vi "ScannerControl.vi"() -> ()   [LabVIEW 2020]
uses:
  <vilib>/Math Plots/3D Math Plots/3D Scatter/3D Scatter XCtrl/3D Scatter.xctl
  <vilib>/userDefined/High Color/IMAQdx.ctl
  <vilib>/vision/Image Controls.llb/IMAQ Image.ctl
  SubVI/GRBL/Status.ctl
  <vilib>/event_ctls.llb/usereventprio.ctl
  <vilib>/vision/driver/IMAQdx.llb/IMAQdx Buffer Number Mode.ctl
  <vilib>/Math Plots/3D Math Plots/3D Scatter/3D Scatter Datatype/Public/Plot Helper (Vector).vi
  <vilib>/Instr/_visa.llb/VISA Configure Serial Port (Instr).vi
  <vilib>/ErrorRing/Error Ring.xnode
  SubVI/GRBL/GRBL 1.1.lvlib
  <vilib>/Math Plots/3D Math Plots/3D Scatter/3D Scatter Datatype/3D Scatter Datatype.lvclass
  <vilib>/vision/driver/NI_Vision_Acquisition_Software.lvlib
panel:
  out "LocationPollingStart":u32
  out "error out":errorcluster
  in  "Save Button":bool
  out "Sys Status":T1
  out "dt polling (ms)":dbl
  out "X encoder count":dbl format="%.2f"
  out "Z Distance(mm)":dbl
  out "X (mm)":dbl
  in  "3DProfileScan":bool
  in  "Pre Scan Speed (mm/min)":sgl=3000.0
  in  "Y Pixel Size(mm)":dbl=1.0
  in  "Y distance(mm)":dbl=10.0
  in  "X distance (mm)":dbl=10.0
  in  "Range Finder COM":refnum<visa-resource-name>="COM5"
  in  "Stage COM port":refnum<visa-resource-name>="COM4"
  in  "ShowFLImIntensity":bool
  in  "Upper Z limite(mm)":dbl=10.0
  in  "Remove Z outlier":bool
  in  "Probe Radius(2mm)":dbl=2.0 format="%#_13g"
  in  "Interpolate Scan":bool
  in  "FollowScanGridSize(mm)":dbl=2.0 format="%#_13g"
  in  "Calc follow scan":bool
  in  "Follow Z offset(mm)":dbl=1.0
  out "3D Profile":refnum<class "3D Plot Datatype.lvclass">[](xcontrol)
  in  "Follow Speed (mm/min)":sgl=3000.0
  in  "Follow Scan":bool
  in  "Plot 3D":bool
  in  "Tab Control":T2(tab)
  out "Scan Origin MPos":cluster{"X":sgl, "Y":sgl, "Z":sgl}
  in  "Set Origin":bool
  in  "Jog Step Size(mm)":dbl=5.0
  in  "Z--":bool
  in  "Z++":bool
  in  "Y--":bool
  in  "Y++":bool
  in  "X--":bool
  in  "X++":bool
  in  "Hault":bool
  in  "Home":bool
  in  "GoToZero":bool
  out "Current Machine Pos":cluster{"X":sgl, "Y":sgl, "Z":sgl}
  in  "Poll grbl position?":bool
  out "Stage Home MPos":cluster{"X":sgl, "Y":sgl, "Z":sgl}
  in  "Stop":bool
  in  "Start":bool
  in  "AccuRangeLoopStopFlag":bool
  out "read buffer":string
  out "Y Graph":dbl[](graph)
  out "X Graph":dbl[](graph)
  out "Z Graph":dbl[](graph)
  in  "X-Axis configuration":T3={"Travel resolution\t(step/mm)"=160.0, "Maximum rate\t(mm/min)"=6000, "Acceleration\t(mm/sec^2)"=1000, "Maximum travel\t(mm)"=100}
  in  "Y-Axis configuration":T3={"Travel resolution\t(step/mm)"=160.0, "Maximum rate\t(mm/min)"=2000, "Acceleration\t(mm/sec^2)"=250, "Maximum travel\t(mm)"=150}
  in  "Z-Axis configuration":T3={"Travel resolution\t(step/mm)"=160.0, "Maximum rate\t(mm/min)"=2000, "Acceleration\t(mm/sec^2)"=250, "Maximum travel\t(mm)"=70}
  out "Current Config":string="$0=10\r\n$1=255\r\n$2=0\r\n$3=0\r\n$4=0\r\n$5=1\r\n$6=0\r\n$10=1\r\n$11=0.010\r\n$12=1000.000\r\n$13=0\r\n$20=1\r\n$21=0\r\n$22=1\r\n$23=0\r\n$24=5.000\r\n$25=3000.000\r\n$26=25\r\n$27=2.000\r\n$30=12000\r\n$31=4000\r\n$32=0\r\n$100=13.333\r\n$101=13.333\r\n$102=98.000\r\n$110=50000.000\r\n$111=50000.000\r\n$112=1800.000\r\n$120=250.000\r\n$121=250.000\r\n$122=50.000\r\n$130=267.000\r\n$131=472.000\r\n$132=68.000\r\nok\r\nok\r\n"
  out "Version information":string="[VER:1.1f.20170324:]\r\n[OPT:VM,15,128]\r\nok\r\nok\r\n"
  in  "CamSession In":T4="cam0"
  out "New Image":T5
  in  "Preview":bool
  out "Image":T5(plugin-control)
  out "PPIX intensity trace":dbl(graph)
  in  "FollowScan":bool
  out "CH1":refnum<class "3D Plot Datatype.lvclass">[](xcontrol)
  out "3D scan":errorcluster
  in  "Quit":bool
  # "Current Position"
  # "3D Profile Scan Setting"
  # "Please wait 5s between start and stop"
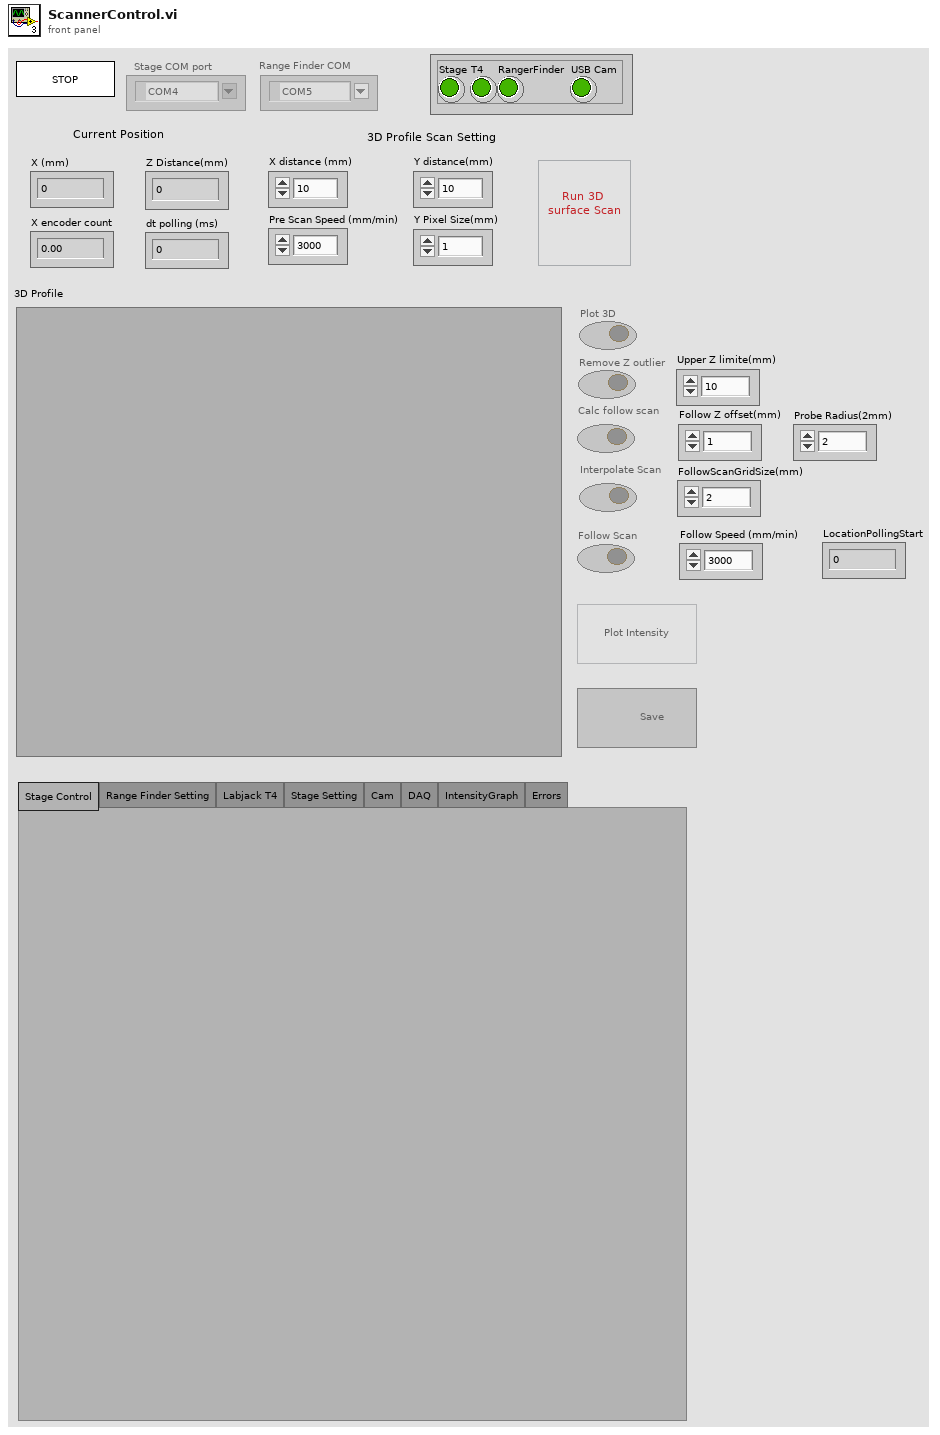
[diagram p1: front panel]
types:
  T1 = cluster{"Stage":bool, "T4":bool, "RangerFinder":bool, "USB Cam":bool}
  T2 = enum32{"Stage Control", "Range Finder Setting", "Labjack T4", "Stage Setting", "Cam", "DAQ", "IntensityGraph", "Errors"}
  T3 = cluster{"Travel resolution\t(step/mm)":sgl, "Maximum rate\t(mm/min)":u32, "Acceleration\t(mm/sec^2)":u32, "Maximum travel\t(mm)":u32}
  T4 = typedef "IMAQdx.ctl" = refnum<k21>
  T5 = typedef "IMAQ Image.ctl" = refnum<image>
  T6 = enum8{"Enabled", "Disabled", "Disabled and Grayed Out"}
  T7 = typedef "NI_Vision_Acquisition_Software.lvlib/IMAQdx Buffer Number Mode.ctl" = enum32{"Next", "Last", "Buffer Number", "Every", "Last New"}
  T8 = typedef "usereventprio.ctl" = enum32{"high priority", "normal priority"}
  T9 = typedef "GRBL 1.1.lvlib/Status.ctl" = enum16{"", "Alarm", "Idle", "Run", "Home"}
  T10 = enum32{"Invalid", "Standard", "Closed", "Hidden", "Minimized", "Maximized"}
  T11 = enum32{"invalid app kind", "Development System", "Run Time System", "Student Edition", "Embedded LabVIEW", "Evaluation", "Custom"}
  T12 = enum16{"open", "open or create", "create or replace", "create", "open (read-only)"}
  T13 = cluster{"Invert enable pin":bool, "Invert limit pin":bool, "Invert probe pin":bool}
  T14 = cluster{"Reverse X":bool, "Reverse Y":bool, "Reverse Z":bool}
  T15 = cluster{"Core":cluster{"Current VI Reference":refnum<vi>, "Close Panel on Exit?":bool}, "Sys Status":cluster{"Stage":bool, "T4":bool, "RangerFinder":bool, "USB Cam":bool}, "StageCOM":refnum<visa-resource-name>, "RangeCOM":refnum<visa-resource-name>, "StepSize":dbl, "ScanOrigin":cluster{"X":sgl, "Y":sgl, "Z":sgl}, "HomeMposOrigin":cluster{"X":sgl, "Y":sgl, "Z":sgl}, "Tic":i32, "IMAQ":T5, "USBCam":T4, "3DProfile":cluster{"x(mm)":dbl, "y(mm)":dbl, "z(mm)":dbl}[], "Raw3DProfile":cluster{"x(mm)":dbl, "y(mm)":dbl, "z(mm)":dbl}[], "FollowScanZOffset(mm)":dbl, "YPixelSize(mm)":dbl, "FollowScanWInter":cluster{"x(mm)":dbl, "y(mm)":dbl, "z(mm)":dbl}[], "BG(V)":dbl, "StageHomed?":bool, "3DProfileToPlot":cluster{"x(mm)":dbl, "y(mm)":dbl, "z(mm)":dbl}[], "FollowScan":cluster{"x(mm)":dbl, "y(mm)":dbl, "z(mm)":dbl}[], "SaveFilePath":path, "Raw3DProfileNoY":cluster{"x(mm)":dbl, "y(mm)":dbl, "z(mm)":dbl}[], "tdms file":refnum<k34>, "FiberOffset":cluster{"x":dbl, "y":dbl}, "RawFollowScanData":cluster{"Time(ms)":dbl, "x":dbl}[], "PPIXProcessedImg":cluster{"x":dbl[], "y":dbl[], "Time(ms)":dbl[]}, "ProbeRadius(mm)":dbl, "FollowGridSize(mm)":dbl}
  T16 = cluster{"remote start event":refnum<user-event>, "remove stop  event":refnum<user-event>}
  T17 = cluster{"Current VI Reference":refnum<vi>, "Close Panel on Exit?":bool}
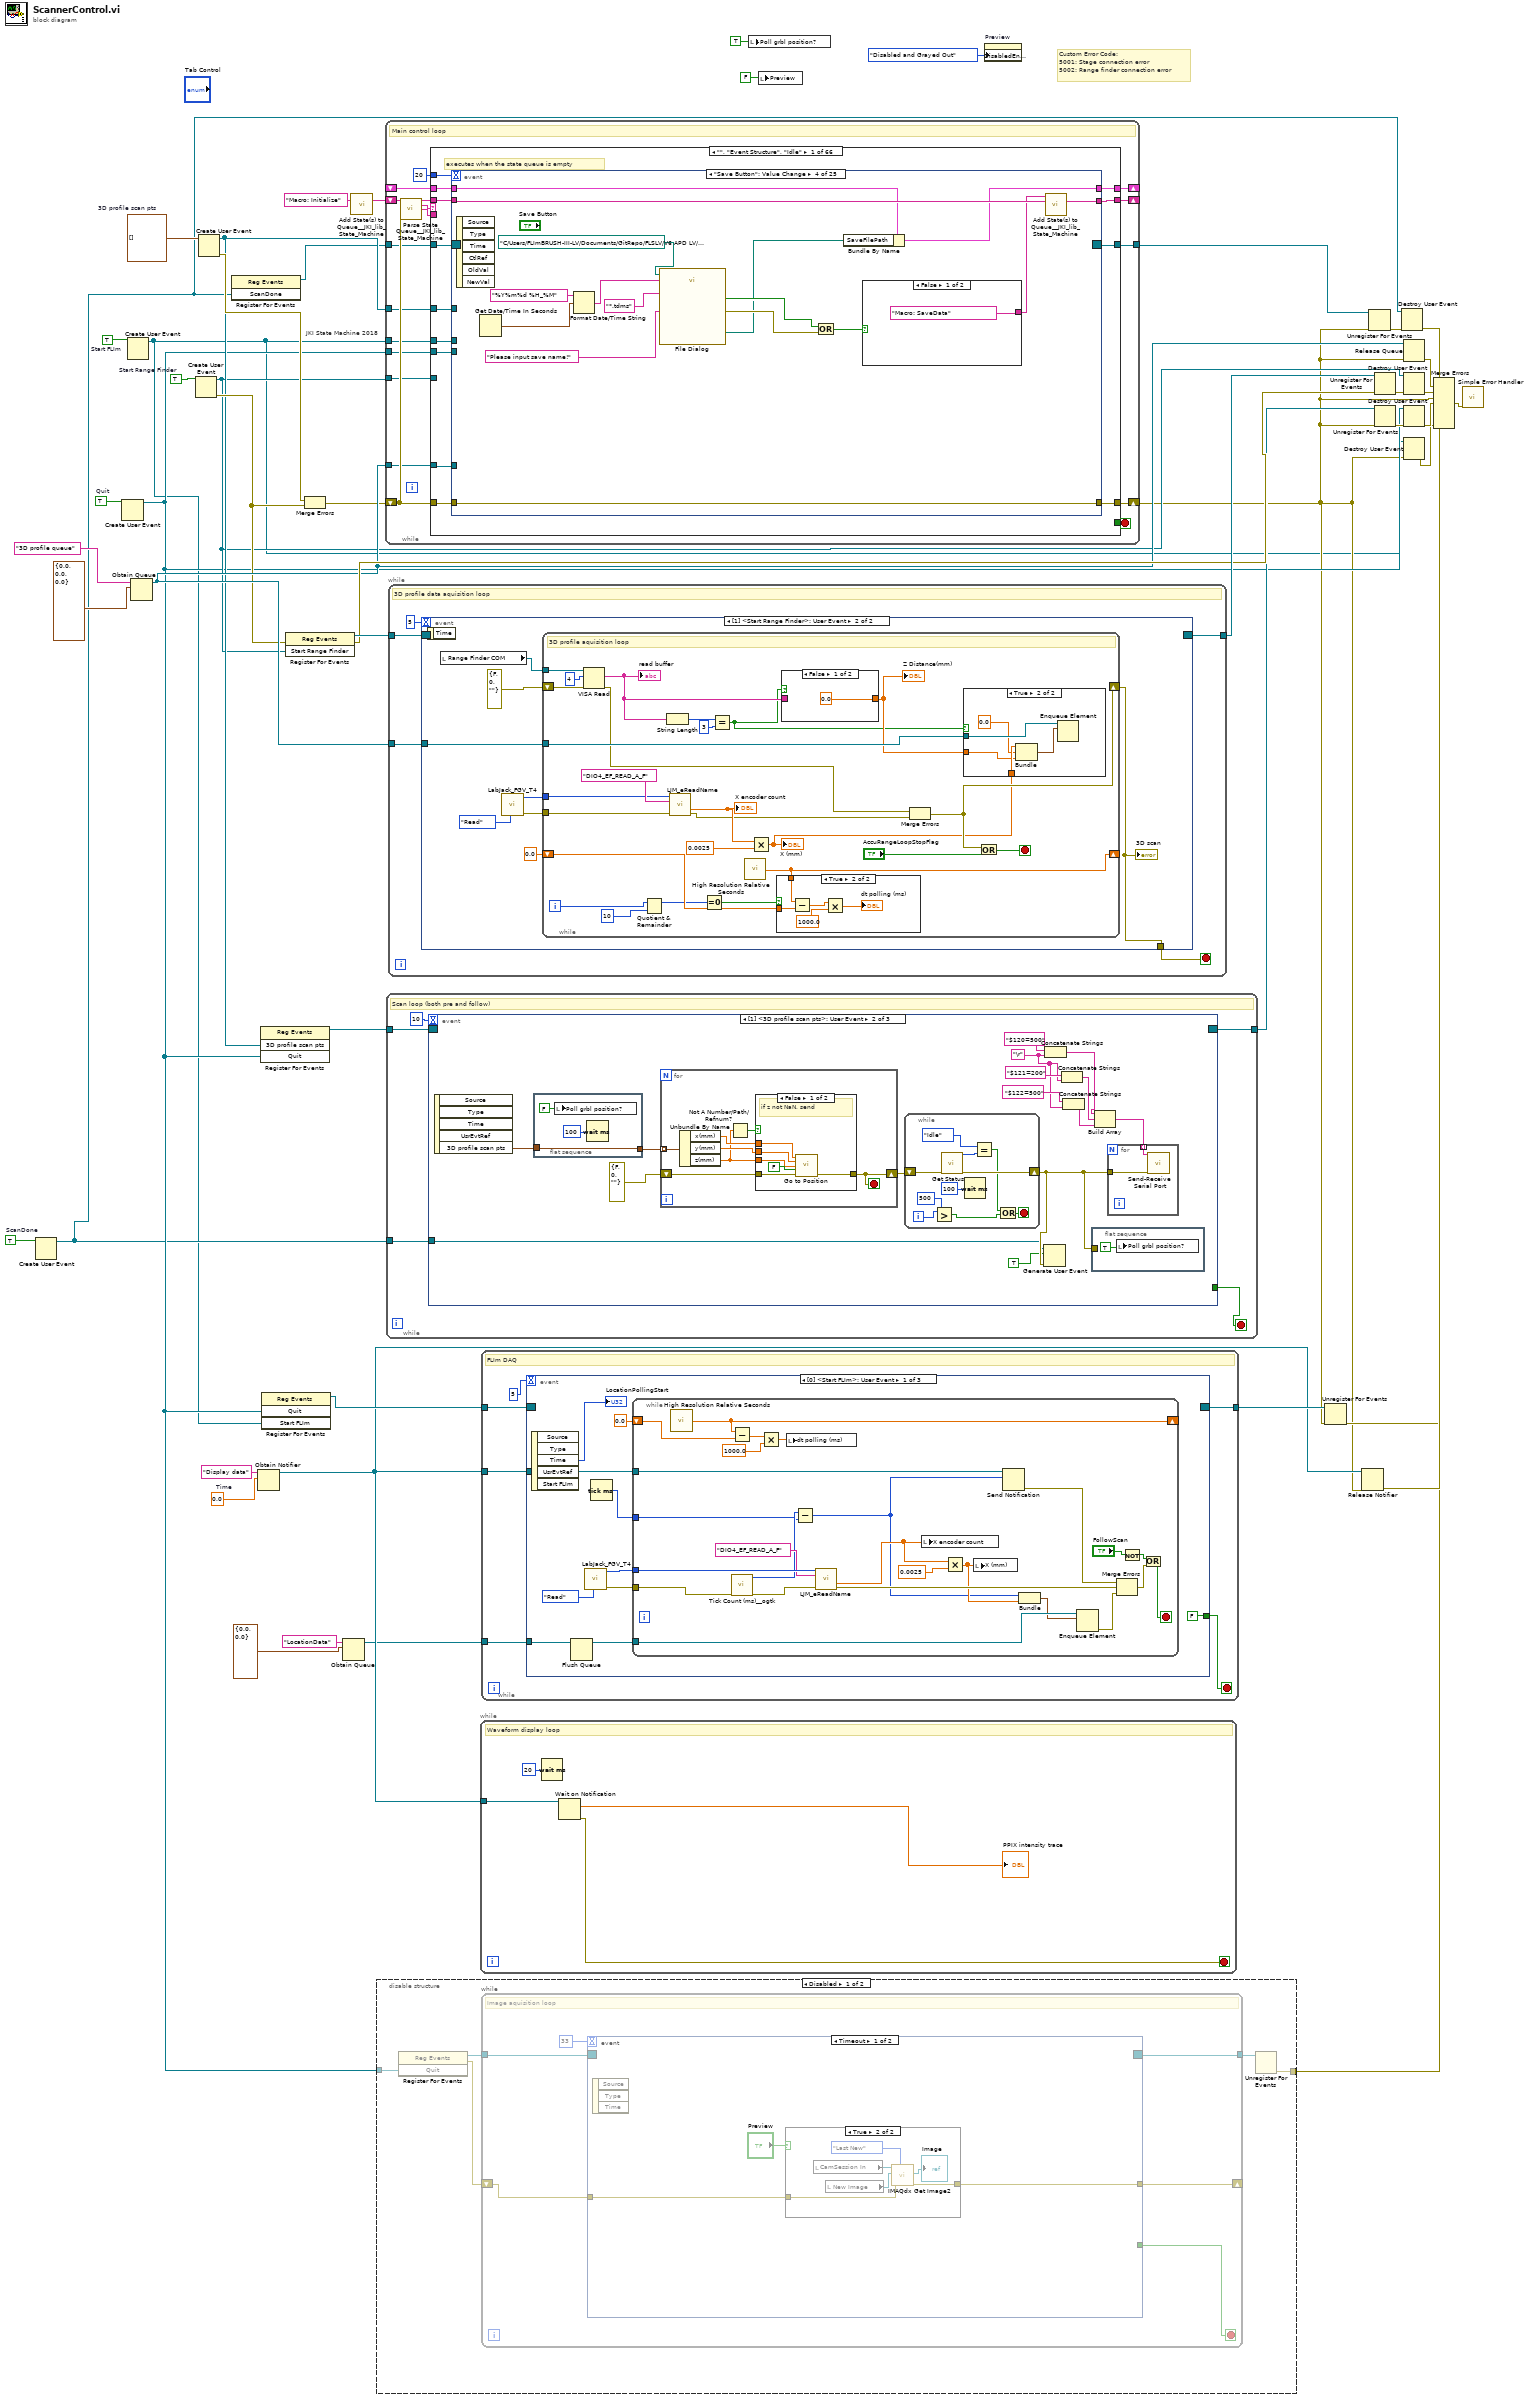
[diagram p0: block diagram]
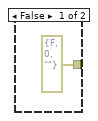
[diagram p2: hidden frame]
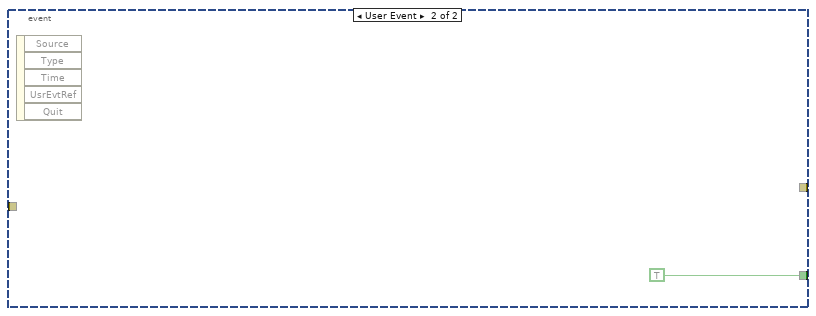
[diagram p3: hidden frame]
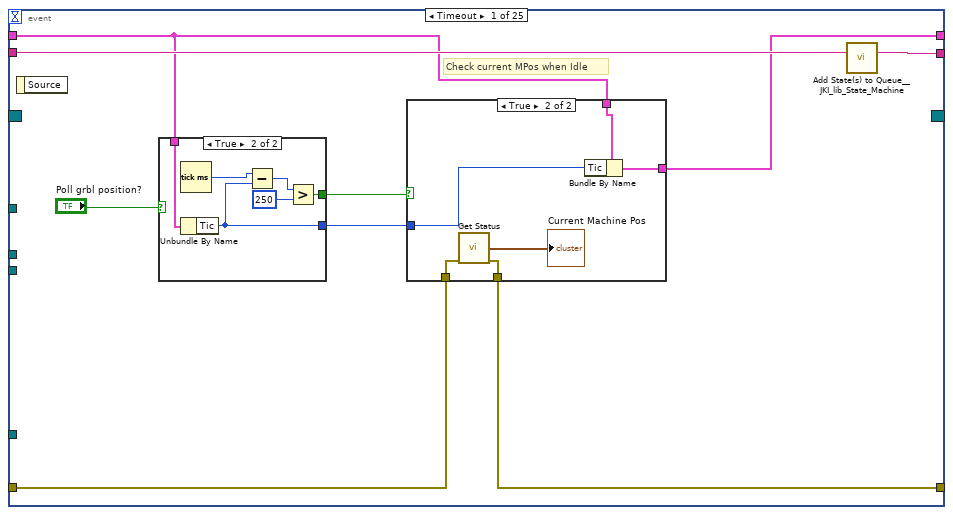
[diagram p5: hidden frame]
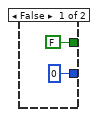
[diagram p6: hidden frame]
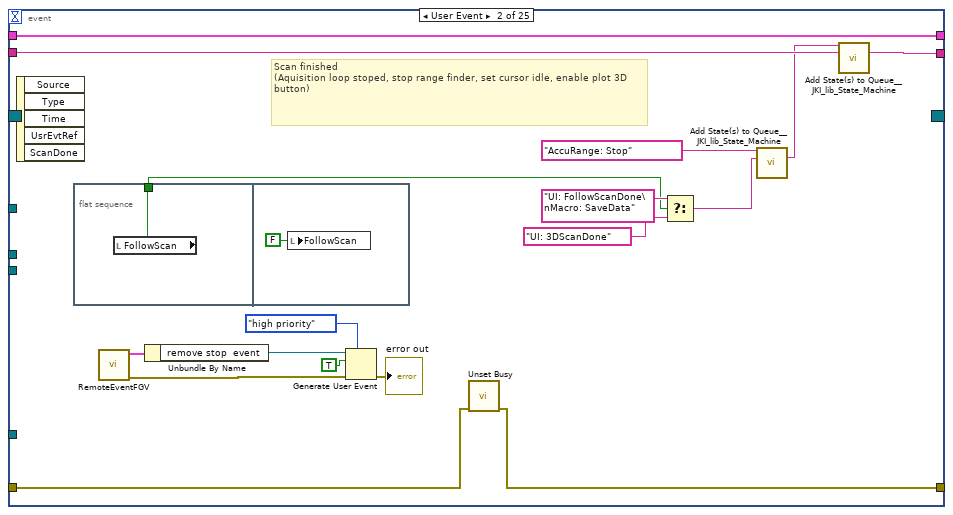
[diagram p8: hidden frame]
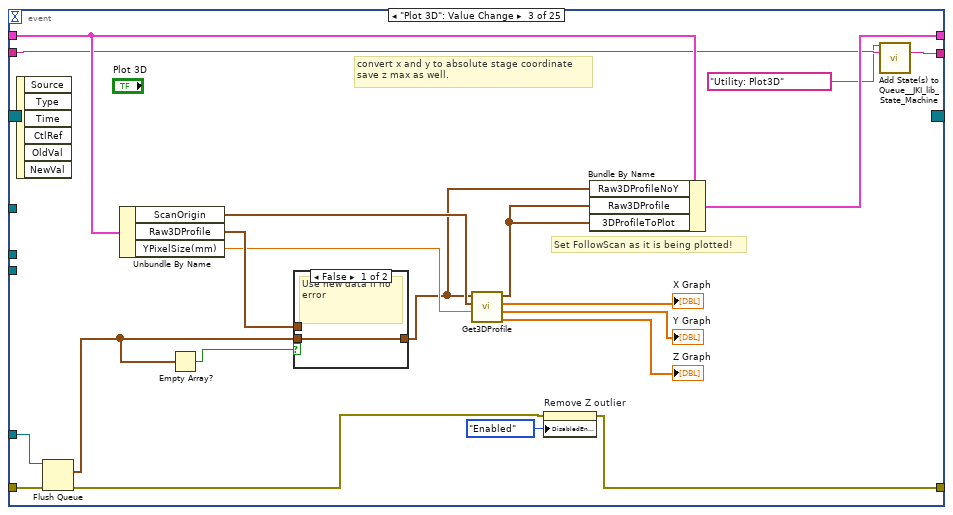
[diagram p9: hidden frame]
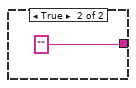
[diagram p11: hidden frame]
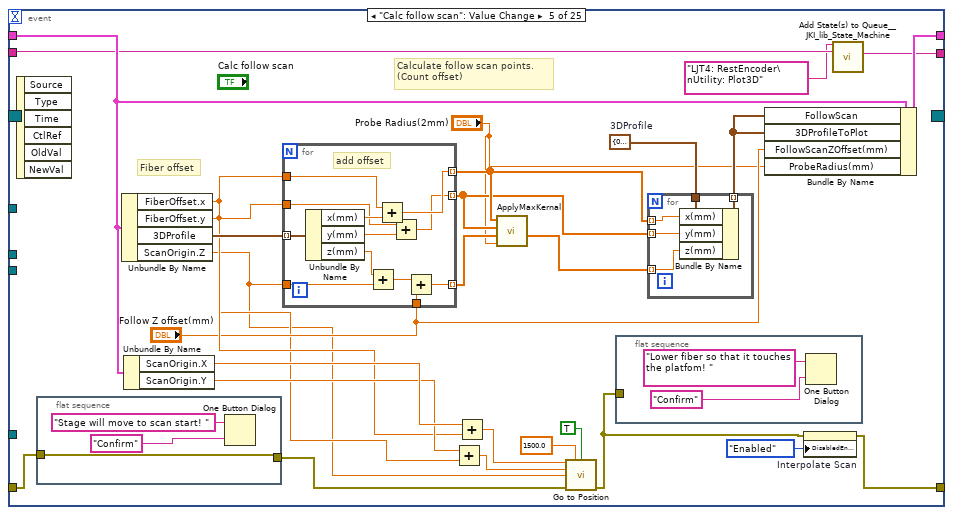
[diagram p12: hidden frame]
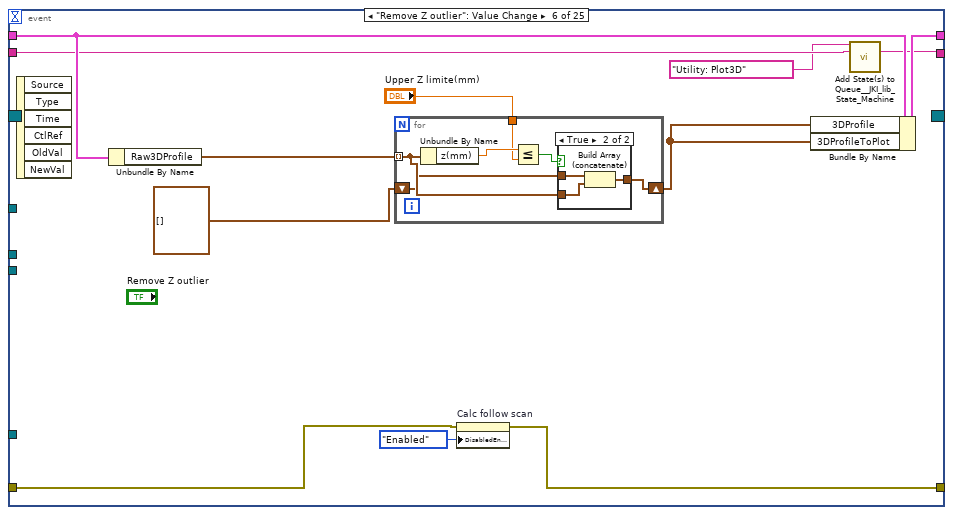
[diagram p13: hidden frame]
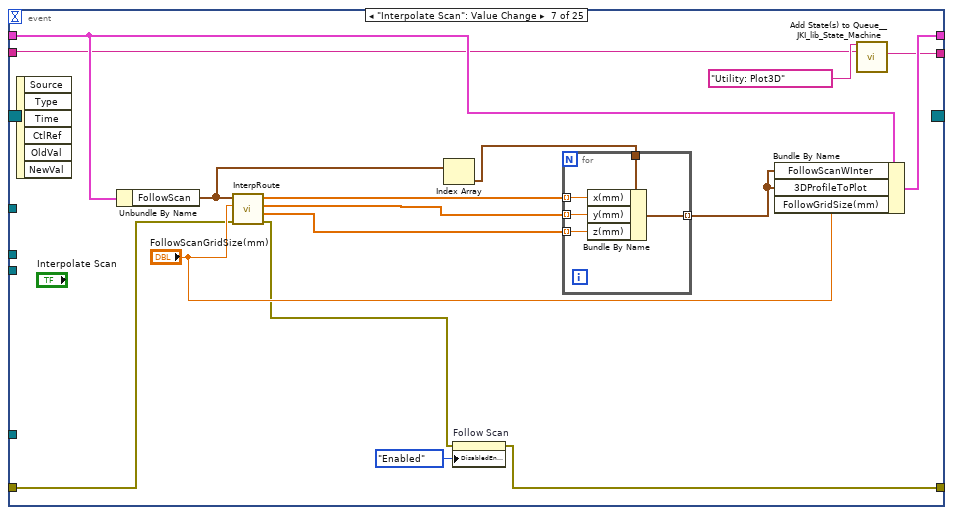
[diagram p15: hidden frame]
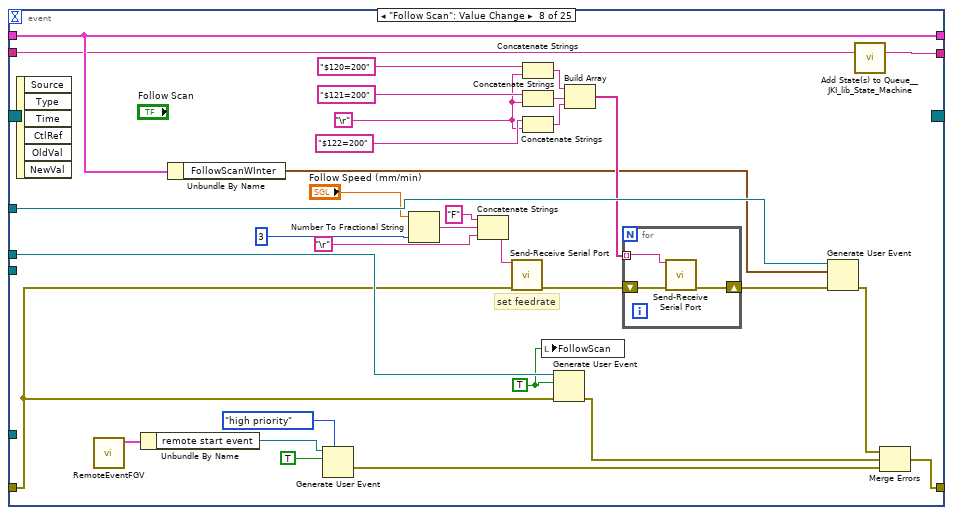
[diagram p16: hidden frame]
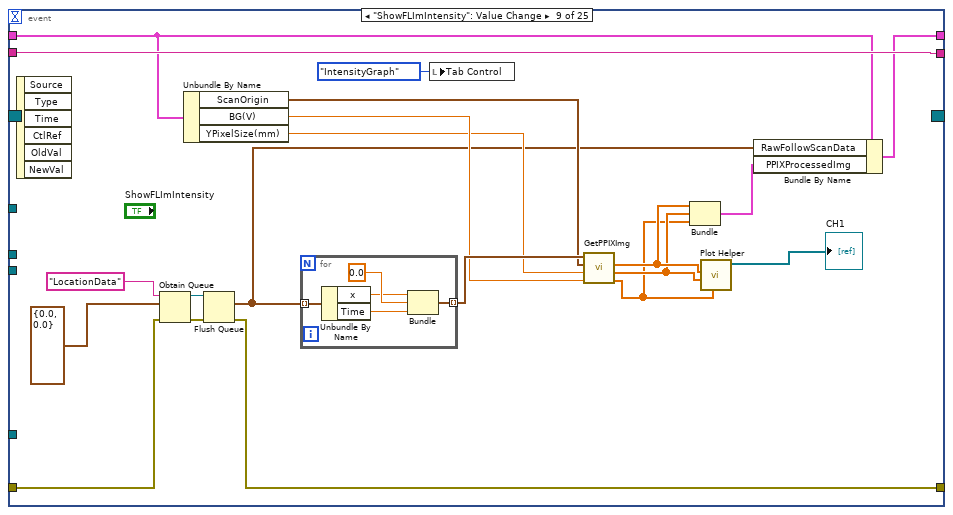
[diagram p17: hidden frame]
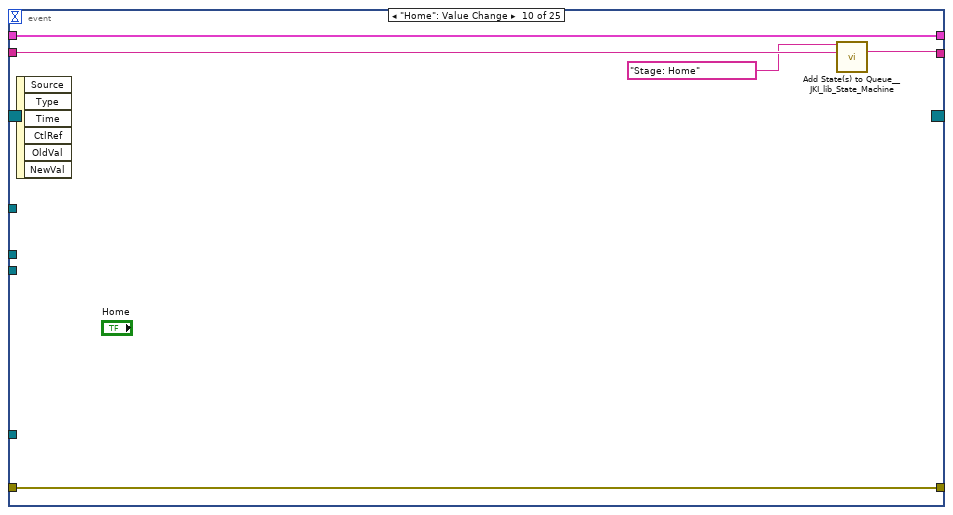
[diagram p18: hidden frame]
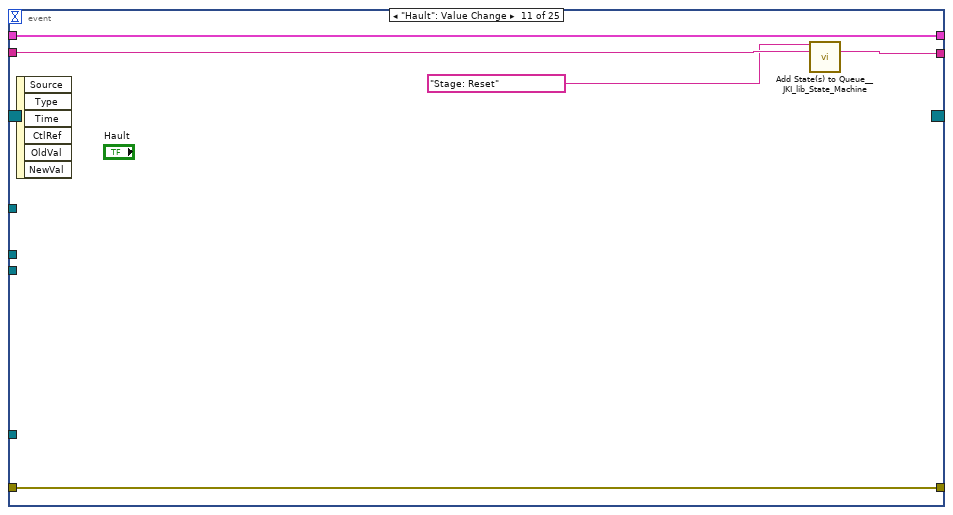
[diagram p19: hidden frame]
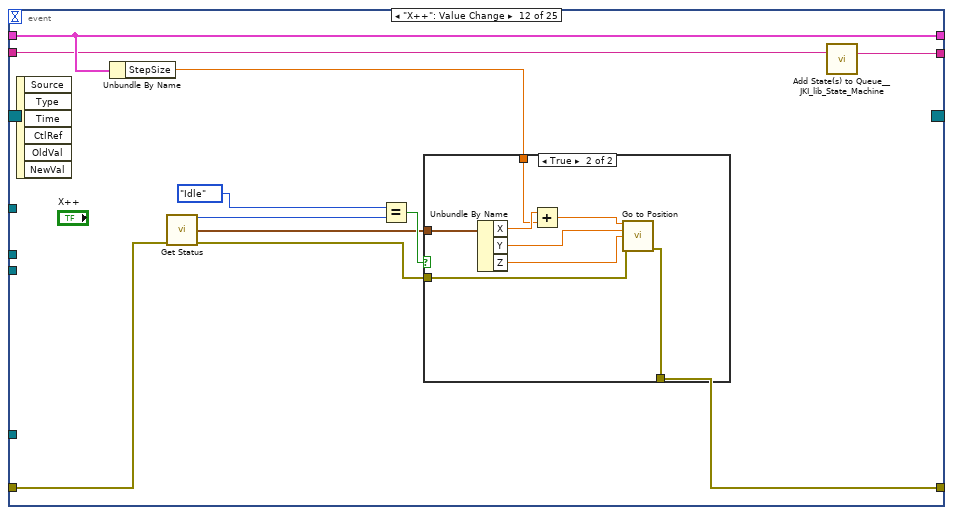
[diagram p20: hidden frame]
diagram:
  w3 = 0.0  # Time
  w12 = TRUE  # ScanDone
  w15 = TRUE  # Start FLIm
  w27 = TRUE  # Quit
  w28 = cluster{"x(mm)":dbl, "y(mm)":dbl, "z(mm)":dbl}[] []  # 3D profile scan pts
  w47 = TRUE  # Start Range Finder
  # "Custom Error Code:\n5001: Stage connection error\n5002: Range finder connection error"
  n1 = Create User Event(user event datatype=w12) -> (user event=w8:refnum<user-event>)  [unwired: 1 in, 1 out]
  n2 = Create User Event(user event datatype=w27) -> (user event=w19:refnum<user-event>)  [unwired: 1 in, 1 out]
  n3 = Create User Event(user event datatype=w15) -> (user event=w1:refnum<user-event>)  [unwired: 1 in, 1 out]
  n4 = Obtain Queue(name (unnamed)="3D profile queue", element data type=cluster{"x(mm)":dbl, "y(mm)":dbl, "z(mm)":dbl} {"x(mm)"=0.0, "y(mm)"=0.0, "z(mm)"=0.0}) -> (queue out=w38:refnum<queue>)  [unwired: 3 in, 2 out]
  n5 = Create User Event(user event datatype=w47) -> (user event=w29:refnum<user-event>, error out=w34:errorcluster)  [unwired: 1 in]
  n6 = Create User Event(user event datatype=w28) -> (user event=w31:refnum<user-event>, error out=w32:errorcluster)  [unwired: 1 in]
  n7 = register-events(w8) -> (reference out=w11:refnum<event-registration>)  [unwired: 2 in, 1 out]
  n8 = Obtain Notifier(name (unnamed)="Display data", notification data type=w3) -> (notifier out=w13:refnum<notifier>)  [unwired: 2 in, 2 out]
  n9 = register-events(w31, w19) -> (reference out=w26:refnum<event-registration>)  [unwired: 2 in, 1 out]
  n10 = register-events(w19, w1) -> (reference out=w22:refnum<event-registration>)  [unwired: 2 in, 1 out]
  n11 = register-events(error in=w34, w29) -> (reference out=w46:refnum<event-registration>, error out=w43:errorcluster)  [unwired: 1 in]
  n12 = Merge Errors(w32, w34) -> (w35:errorcluster)
  n13 = Obtain Queue(name (unnamed)="LocationData", element data type=cluster{"Time":dbl, "x":dbl} {"Time"=0.0, "x"=0.0}) -> (queue out=w4:refnum<queue>)  [unwired: 3 in, 2 out]
  n14 = call <vilib>:"Add State(s) to Queue__JKI_lib_State_Machine.vi"("State(s) in (\"\")"="Macro: Initialize") -> ("States Out"=w49:string)  [unwired: 14 in]
  n15 = disable-structure shown="Disabled" {
    disable-tunnel: w19 -> [w54 _]
    disable-tunnel: [w53 _] -> w18
    frame Disabled {
      n16 = register-events(w54) -> (reference out=w52:refnum<event-registration>, error out=w51:errorcluster)  [unwired: 2 in]
      n17 = while {
        shift-right: [w59] -> _
        shift-left: w51 -> [w58]
        tunnel: w52 -> [w57]
        tunnel: [w55] -> w50
        stop <- w56 stop-if-true
        # "Image aquisition loop"
        n18 = event shown="[0] Timeout" {
          selector: w57 -> [_ _]
          dyn-events: [_ _] -> w55
          timeout: u32 33 ("milliseconds to wait") -> [_ _]
          tunnel: [w62 _] -> w59
          tunnel: w58 -> [w61 _]
          tunnel: [_ TRUE] -> w56
          event Timeout {
            n19 = event-data() -> ()  [unwired: 1 in, 3 out]
            n20 = case shown="True" "Preview" {
              tunnel: [errorcluster {"status"=FALSE, "code"=0, "source"=""} ("error out") w66] -> w62
              tunnel: w61 -> [_ w65]
              frame False {
              }
              frame True {
                n21 = local read "CamSession In"() -> (w68:T4)
                n22 = local read "New Image"() -> (w69:T5)
                n23 = call <vilib>:"IMAQdx Get Image2.vi"("Buffer Number Mode (Next)"=IMAQdx_Buffer_Number_Mode."Last New", "error in"=w65, "Image In"=w69, "Session In"=w68) -> ("error out"=w66:errorcluster, "Image Out"=→"Image":T5)  [unwired: 4 in, 2 out]
              }
            }
          }
          event User Event {
            n24 = event-data() -> ()  [unwired: 1 in, 5 out]
          }
        }
      }
      n25 = Unregister For Events(event registration refnum=w50) -> (error out=w53:errorcluster)  [unwired: 1 in]
    }
    frame Enabled {
    }
  }
  n26 = while "JKI State Machine 2018" {
    shift-right: [w84] -> _
    shift-left: _ -> [w72]
    shift-right: [w87] -> w9
    shift-left: w35 -> [w82]
    shift-right: [w86] -> _
    shift-left: w49 -> [w80]
    tunnel: w29 -> [w81]
    tunnel: w38 -> [w79]
    tunnel: w31 -> [w78]
    tunnel: w19 -> [w77]
    tunnel: w1 -> [w76]
    tunnel: w11 -> [w74]
    tunnel: [w73] -> w10
    stop <- w85 stop-if-true
    # "Main control loop"
    n27 = call <vilib>:"Parse State Queue__JKI_lib_State_Machine.vi"("State Queue"=w80, "Error In (no error)"=w82) -> ("Remaining States"=w89:string, "Current State"=w75:string, "Arguments"=w88:string)  [unwired: 11 in]
    n28 = case shown="\"\", \"Event Structure\", \"Idle\"" w75 {
      selector: w75 -> [_ _ _ _ _ _ w576 _ _ _ _ _ _ _ _ _ _ _ _ _ _ _ _ _ _ _ _ _ _ _ _ _ _ _ _ _ _ _ _ _ _ _ _ _ _ _ _ _ _ _ _ _ _ _ _ _ _ _ _ _ _ _ _ _ _ _]
      tunnel: w89 -> [w102 w545 w551 w552 w569 w574 w580 w600 w607 w616 w621 w653 w660 w667 w688 w701 w729 w751 w792 w820 w852 w869 w876 w892 w903 w909 w916 w923 w929 w934 w942 w949 w956 w968 w1038 w1050 w1068 w1099 w1110 w1133 w1179 w1187 w1199 w1215 w1247 w1271 w1284 w1304 w1319 w1329 w1339 w1350 w1355 w1367 w1377 w1395 w1403 w1418 w1435 w1450 w1460 w1475 w1484 w1489 w1494 w1499]
      tunnel: w88 -> [_ _ _ _ _ _ _ _ _ _ _ _ _ _ _ _ _ _ _ _ _ _ _ _ _ _ _ _ _ _ _ _ w951 w962 _ _ _ _ _ _ w1174 _ _ _ _ _ _ _ _ _ _ w1346 _ _ _ _ _ _ _ _ _ _ _ _ _ _]
      tunnel: w72 -> [w100 w542 w548 w555 w566 w571 w578 w593 w604 w614 w618 _ w656 w662 w682 w698 w726 w748 w789 w817 w849 w866 w873 w883 w900 w906 w913 w920 w926 w931 w939 w947 w954 w964 w1035 w1040 w1066 w1080 w1106 w1127 w1177 w1181 w1196 w1209 w1245 w1268 w1282 w1297 w1316 w1327 w1335 w1347 w1352 w1362 w1375 w1393 w1397 w1415 w1429 w1443 w1453 w1472 w1480 w1486 w1491 w1496]
      tunnel: [w99 w543 w549 w556 w567 w572 w582 w597 errorcluster {"status"=FALSE, "code"=0, "source"=""} ("error out") w610 w619 w650 w658 w663 w684 w691 w702 w736 w756 w797 w828 w860 w871 w878 w901 w907 w914 w921 w927 w932 w940 w946 w952 w965 w1036 w1044 w1065 w1074 w1108 w1130 w1176 w1185 w1197 w1200 w1229 w1263 w1278 w1301 w1317 w1322 w1337 w1348 w1353 w1364 w1369 w1380 w1401 w1416 w1428 w1446 w1457 w1473 w1482 w1487 w1492 w1497] -> w87
      tunnel: w82 -> [w98 w543 w549 w556 w567 w572 w581 w597 w603 w609 w619 w650 w658 w664 w683 w696 w709 w735 w777 w805 w842 w862 w870 w877 w901 w907 w914 w921 w927 w932 w940 w946 w953 w966 w1036 w1048 w1064 w1079 w1104 w1131 w1175 w1184 w1197 w1211 w1230 w1261 w1280 w1300 w1317 w1321 w1337 w1348 w1353 w1360 w1368 w1379 w1400 w1416 w1430 w1445 w1456 w1473 w1482 w1487 w1492 w1497]
      tunnel: [w101 w544 w550 w557 w568 w573 w579 w599 w606 w615 w620 w652 w659 w666 w687 w700 w728 w750 w791 w819 w851 w868 w875 w891 w902 w908 w915 w922 w928 w933 w941 w948 w955 w967 w1037 w1049 w1067 w1098 w1109 w1132 w1178 w1186 w1198 w1214 w1246 w1270 w1283 w1303 w1318 w1328 w1338 w1349 w1354 w1366 w1376 w1394 w1402 w1417 w1434 w1449 w1459 w1474 w1483 w1488 w1493 w1498] -> w86
      tunnel: [_ _ _ _ _ _ _ _ _ TRUE _ _ _ _ _ _ _ _ _ _ _ _ _ _ _ _ _ _ _ _ _ _ _ _ _ _ _ _ _ _ _ _ _ _ _ _ _ _ _ _ _ _ _ _ _ _ _ _ _ _ _ _ _ _ _ _] -> w85
      tunnel: [w97 w542 w548 w555 w566 w571 w578 w598 w604 w614 w618 w651 w657 w662 w681 w698 w726 w748 w789 w817 w849 w866 w873 w882 w900 w906 w913 w920 w926 w931 w939 w947 w954 w964 w1035 w1047 w1066 w1080 w1107 w1129 w1177 w1182 w1196 w1208 w1245 w1268 w1282 w1298 w1316 w1327 w1335 w1347 w1352 w1363 w1375 w1393 w1398 w1415 w1426 w1443 w1454 w1472 w1480 w1486 w1491 w1496] -> w84
      tunnel: 20 ("Timeout") -> [w96 _ _ _ _ _ _ _ _ _ _ _ _ _ _ _ _ _ _ _ _ _ _ _ _ _ _ _ _ _ _ _ _ _ _ _ _ _ _ _ _ _ _ _ _ _ _ _ _ _ _ _ _ _ _ _ _ _ _ _ _ _ _ _ _ _]
      tunnel: w81 -> [_ _ _ _ _ _ _ _ _ _ _ _ _ _ _ _ _ _ _ _ _ _ _ _ _ _ _ _ _ _ _ _ _ _ _ _ _ _ _ _ _ _ _ _ _ w1267 _ _ _ _ _ _ _ _ _ _ _ _ _ _ _ _ _ _ _ _]
      tunnel: w79 -> [w95 _ _ _ _ _ _ _ _ _ _ _ _ _ _ _ _ _ _ _ _ _ _ _ _ _ _ _ _ _ _ _ _ _ _ _ _ _ _ _ _ _ _ _ _ _ _ _ _ _ _ _ _ _ _ _ _ _ _ _ _ _ _ _ _ _]
      tunnel: w78 -> [w94 _ _ _ _ _ _ _ _ _ _ _ _ _ _ _ _ _ _ _ _ _ _ _ _ _ _ _ _ _ _ _ _ _ _ _ _ _ _ _ _ _ _ _ _ _ _ _ _ _ _ _ _ _ _ _ _ _ _ _ _ _ _ _ _ _]
      tunnel: w77 -> [w93 _ _ _ _ _ _ _ _ w611 _ _ _ _ _ _ _ _ _ _ _ _ _ _ _ _ _ _ _ _ _ _ _ _ _ _ _ _ _ _ _ _ _ _ _ _ _ _ _ _ _ _ _ _ _ _ _ _ _ _ _ _ _ _ _ _]
      tunnel: w76 -> [w92 _ _ _ _ _ _ _ _ _ _ _ _ _ _ _ _ _ _ _ _ _ _ _ _ _ _ _ _ _ _ _ _ _ _ _ _ _ _ _ _ _ _ _ _ _ _ _ _ _ _ _ _ _ _ _ _ _ _ _ _ _ _ _ _ _]
      tunnel: w74 -> [w91 w541 w547 w553 w558 w570 w575 w587 w601 w608 w617 w633 w654 w661 w686 w699 w727 w749 w790 w818 w850 w867 w874 w890 w899 w905 w912 w919 w925 w930 w938 w945 w950 w961 w1034 w1042 w1063 w1070 w1105 w1128 w1173 w1180 w1195 w1201 w1228 w1248 w1274 w1296 w1315 w1326 w1330 w1344 w1351 w1361 w1374 w1378 w1396 w1414 w1419 w1441 w1452 w1471 w1481 w1485 w1490 w1495]
      tunnel: [w90 w541 w547 w553 w558 w570 w575 w587 w601 w608 w617 w633 w654 w661 w686 w699 w727 w749 w790 w818 w850 w867 w874 w890 w899 w905 w912 w919 w925 w930 w938 w945 w950 w961 w1034 w1042 w1063 w1070 w1105 w1128 w1173 w1180 w1195 w1201 w1228 w1248 w1274 w1296 w1315 w1326 w1330 w1344 w1351 w1361 w1374 w1378 w1396 w1414 w1419 w1441 w1452 w1471 w1481 w1485 w1490 w1495] -> w73
      frame "", "Event Structure", "Idle" {
        # "executes when the state queue is empty"
        n29 = event shown="[3] \"Save Button\": Value Change" {
          selector: w91 -> [_ _ _ _ _ _ _ _ _ _ _ _ _ _ _ _ _ _ _ _ _ _ _ _ _]
          dyn-events: [_ _ _ _ _ _ _ _ _ _ _ _ _ _ _ _ _ _ _ _ _ _ _ _ _] -> w90
          timeout: w96 -> [_ _ _ _ _ _ _ _ _ _ _ _ _ _ _ _ _ _ _ _ _ _ _ _ _]
          tunnel: w102 -> [w111 w142 w160 w182 w202 w244 w265 w291 w328 w342 w348 w358 w379 w393 w405 w426 w447 w467 w490 w502 w517 w524 w528 w533 w540]
          tunnel: [w110 w143 w159 w183 w203 w243 w264 w292 w328 w343 w347 w359 w380 w394 w406 w427 w448 w467 w489 w503 w517 w523 w527 w532 w539] -> w101
          tunnel: w100 -> [w105 w144 w163 w175 w212 w246 w272 w311 w320 w344 w349 w360 w381 w396 w407 w428 w449 w470 w478 w504 w519 w522 w529 w534 w537]
          tunnel: [w109 w130 w149 w184 w205 w239 w267 w287 w329 w341 w345 w351 w372 w395 w398 w419 w440 w460 w471 w495 w515 w520 w525 w530 w538] -> w99
          tunnel: w98 -> [w108 w132 w165 w184 w200 w238 w260 w289 w331 w341 w345 w350 w371 w395 w397 w418 w439 w465 w487 w494 w515 w520 w525 w530 w538]
          tunnel: [w106 w144 w164 w174 w213 w245 w271 w311 w321 w344 w349 w360 w381 w396 w407 w428 w449 w469 w479 w504 w518 w522 w529 w534 w537] -> w97
          tunnel: w95 -> [_ _ w166 _ _ _ _ _ _ _ _ _ _ _ _ _ _ _ w488 _ _ _ _ _ _]
          tunnel: w94 -> [_ _ _ _ _ _ _ w310 _ _ _ _ _ _ _ _ _ _ w476 _ _ _ _ _ _]
          tunnel: w93 -> [_ _ _ _ _ _ _ _ _ _ _ _ _ _ _ _ _ _ _ _ _ _ _ _ _]
          tunnel: w92 -> [_ _ _ _ _ _ _ w290 _ _ _ _ _ _ _ _ _ _ _ _ _ _ _ _ _]
          event Timeout {
            # "Check current MPos when Idle"
            n30 = event-data() -> ()  [unwired: 1 in, 1 out]
            n31 = case shown="True" "Poll grbl position?" {
              tunnel: [FALSE w116] -> w107
              tunnel: w105 -> [_ w115]
              tunnel: [0 ("Tic") w114] -> w104
              frame False {
              }
              frame True {
                n32 = Tick Count (ms)() -> (millisecond timer value=w119:u32)
                n33 = Unbundle By Name(w115) -> ("Tic"=w114:i32)
                n34 = Subtract(x=w119, y=w114) -> (x-y=w118:u32)
                n35 = Greater?(x=w118, y=u32 250) -> (0:w116:bool)
              }
            }
            n36 = case shown="True" w107 {
              tunnel: [w121 w127] -> w109
              tunnel: w108 -> [w121 w126]
              tunnel: w105 -> [w120 w124]
              tunnel: [w120 w123] -> w106
              tunnel: w104 -> [_ w122]
              frame False {
              }
              frame True {
                n37 = call "Get Status.vi"("error in (no error)"=w126) -> ("Current position"=→"Current Machine Pos":cluster{"X":sgl, "Y":sgl, "Z":sgl}, "error out"=w127:errorcluster)  [unwired: 10 in, 3 out]
                n38 = Bundle By Name(cluster=w124, "Tic"=w122) -> (w123:T15)
              }
            }
            n39 = call <vilib>:"Add State(s) to Queue__JKI_lib_State_Machine.vi"("State(s) in (\"\")"=w111) -> ("States Out"=w110:string)  [unwired: 14 in]
          }
          event User Event {
            # "Scan finished\n(Aquisition loop stoped, stop range finder, set cursor idle, enable plot 3D button)"
            n40 = event-data() -> ()  [unwired: 1 in, 5 out]
            n41 = flat-sequence {
              tunnel: [w145] -> w139
              frame #0 {
                n42 = local read "FollowScan"() -> (w145:bool)
              }
              frame #1 {
                n43 = local write "FollowScan"(FALSE ("InScan")) -> ()
              }
            }
            n44 = call "RemoteEventFGV.vi"() -> ("Error Out"=w131:errorcluster, "Remote Event out"=w135:T16)  [unwired: 10 in]
            n45 = Unbundle By Name(w135) -> ("remove stop  event"=w134:refnum<user-event>)
            n46 = Generate User Event(priority (normal)=usereventprio."high priority", user event=w134, event data cluster=TRUE ("event data"), error in=w131) -> (error out=→"error out":errorcluster)  [unwired: 1 out]
            n47 = call <vilib>:"Unset Busy.vi"("error in (no error)"=w132) -> ("error out"=w130:errorcluster)  [unwired: 10 in]
            n48 = Select(t="UI: FollowScanDone\nMacro: SaveData", s=w139, f="UI: 3DScanDone" ("State(s) in (\"\")")) -> (s? t:f=w137:string)
            n49 = call <vilib>:"Add State(s) to Queue__JKI_lib_State_Machine.vi"("State(s) in Front (\"\")"="AccuRange: Stop" ("State(s) in (\"\")"), "State(s) in (\"\")"=w137) -> ("States Out"=w136:string)  [unwired: 13 in]
            n50 = call <vilib>:"Add State(s) to Queue__JKI_lib_State_Machine.vi"("State(s) in Front (\"\")"=w136, "State(s) in (\"\")"=w142) -> ("States Out"=w143:string)  [unwired: 13 in]
          }
          event "Plot 3D": Value Change {
            # "Set FollowScan as it is being plotted!"
            # "convert x and y to absolute stage coordinate\nsave z max as well."
            n51 = event-data() -> ()  [unwired: 1 in, 6 out]
            n52 = Flush Queue(queue=w166, error in (no error)=w165) -> (remaining elements=w154:cluster{"x(mm)":dbl, "y(mm)":dbl, "z(mm)":dbl}[], error out=w150:errorcluster)  [unwired: 1 out]
            n53 = Unbundle By Name(w163) -> ("ScanOrigin"=w162:cluster{"X":sgl, "Y":sgl, "Z":sgl}, "Raw3DProfile"=w157:cluster{"x(mm)":dbl, "y(mm)":dbl, "z(mm)":dbl}[], "YPixelSize(mm)"=w156:dbl)
            n54 = Empty Array?(array=w154) -> (empty?=w153:bool)
            n55 = case shown="False" w153 {
              tunnel: w154 -> [w167 _]
              tunnel: [w167 w168] -> w147
              tunnel: w157 -> [_ w168]
              frame False {
                # "Use new data if no error"
              }
              frame True {
                # "Use old data if error"
              }
            }
            n56 = call "Get3DProfile.vi"("dy"=w156, "Origin"=w162, "remaining elements"=w147) -> ("Z"=→"Z Graph":dbl[], "Y"=→"Y Graph":dbl[], "X"=→"X Graph":dbl[], "3D Profile"=w151:cluster{"x(mm)":dbl, "y(mm)":dbl, "z(mm)":dbl}[])  [unwired: 5 in]
            n57 = property on="Remove Z outlier" class="Bool"(error in=w150, "DisabledEnum"=T6."Enabled" ("Disabled")) -> (error out=w149:errorcluster)  [unwired: 1 in, 1 out]
            n58 = Bundle By Name(cluster=w163, "Raw3DProfileNoY"=w147, "Raw3DProfile"=w151, "3DProfileToPlot"=w151) -> (w164:T15)
            n59 = call <vilib>:"Add State(s) to Queue__JKI_lib_State_Machine.vi"("State(s) in Front (\"\")"="Utility: Plot3D" ("State(s) in Front (\"\")"), "State(s) in (\"\")"=w160) -> ("States Out"=w159:string)  [unwired: 13 in]
          }
          event "Save Button": Value Change {
            n60 = event-data() -> ()  [unwired: 1 in, 6 out]
            n61 = Get Date/Time In Seconds() -> (seconds since 1Jan1904=w171:timestamp)
            n62 = Format Date/Time String(time format string (%c)="%Y%m%d %H_%M", seconds (now)=w171) -> (date/time string=w169:string)  [unwired: 1 in]
            n63 = call "File Dialog"("start path"=path "C:/Users/FLImBRUSH-III-LV/Documents/GitRepo/FLSLV/V6 APD LV/Data", "prompt"="Please input save name!", "default name"=w169, "pattern (all files)"="*.tdms") -> ("selected path"=w173:path, "cancelled"=w178:bool, "error out"=w177:errorcluster)  [unwired: 8 in, 1 out]
            n64 = Or(x=w178, y=w177) -> (x .or. y?=w176:bool)
            n65 = Bundle By Name(cluster=w175, "SaveFilePath"=w173) -> (w174:T15)
            n66 = case shown="False" w176 {
              tunnel: ["Macro: SaveData" ("State(s) in Front (\"\")") "" ("State(s) in Front (\"\")")] -> w179
              frame False {
              }
              frame True {
              }
            }
            n67 = call <vilib>:"Add State(s) to Queue__JKI_lib_State_Machine.vi"("State(s) in Front (\"\")"=w179, "State(s) in (\"\")"=w182) -> ("States Out"=w183:string)  [unwired: 13 in]
          }
          event "Calc follow scan": Value Change {
            w192 = cluster{"x(mm)":dbl, "y(mm)":dbl, "z(mm)":dbl} {"x(mm)"=0.0, "y(mm)"=0.0, "z(mm)"=0.0}  # 3DProfile
            # "Fiber offset"
            # "Calculate follow scan points.\n(Count offset)"
            n68 = event-data() -> ()  [unwired: 1 in, 6 out]
            n69 = flat-sequence {
              tunnel: w200 -> [w222]
              tunnel: [w222] -> w199
              frame #0 {
                n70 = One Button Dialog(message="Stage will move to scan start! ", button name ("OK")="Confirm") -> ()  [unwired: 1 out]
              }
            }
            n71 = Unbundle By Name(w212) -> ("FiberOffset.x"=w197:dbl, "FiberOffset.y"=w189:dbl, "3DProfile"=w214:cluster{"x(mm)":dbl, "y(mm)":dbl, "z(mm)":dbl}[], "ScanOrigin.Z"=w188:sgl)
            n72 = Unbundle By Name(w212) -> ("ScanOrigin.X"=w211:sgl, "ScanOrigin.Y"=w206:sgl)
            n73 = for {
              tunnel: w214 -> [w236] mode=indexing
              tunnel: w188 -> [w235]
              tunnel: "Follow Z offset(mm)" -> [w233]
              tunnel: w197 -> [w229]
              tunnel: w189 -> [w228]
              tunnel: [w227] -> w193 mode=indexing
              tunnel: [w226] -> w191 mode=indexing
              tunnel: [w225] -> w195 mode=indexing
              # "add offset"
              n74 = Unbundle By Name(w236) -> ("x(mm)"=w232:dbl, "y(mm)"=w231:dbl, "z(mm)"=w230:dbl)
              n75 = Add(x=w230, y=w235) -> (x+y=w234:dbl)
              n76 = Add(x=w229, y=w232) -> (x+y=w227:dbl)
              n77 = Add(x=w228, y=w231) -> (x+y=w226:dbl)
              n78 = Add(x=w234, y=w233) -> (x+y=w225:dbl)
            }
            n79 = Add(x=w206, y=w189) -> (x+y=w209:dbl)
            n80 = Add(x=w211, y=w197) -> (x+y=w210:dbl)
            n81 = call "ApplyMaxKernal.vi"("Radius(2mm)"="Probe Radius(2mm)", "Z"=w195, "Y"=w191, "X"=w193) -> ("ZZ"=w194:dbl[])  [unwired: 7 in]
            n82 = call "Go to Position.vi"("X (mm)"=w210, "Speed (2000 mm/min)"=sgl 1500.0 ("Speed (mm/min)"), "Overwright speed? (F)"=TRUE, "Y (mm)"=w209, "Z (mm)"=w188, "error in (no error)"=w199) -> ("error out"=w198:errorcluster)  [unwired: 9 in]
            n83 = flat-sequence {
              tunnel: w198 -> [_]
              frame #0 {
                n84 = One Button Dialog(message="Lower fiber so that it touches the platfom! ", button name ("OK")="Confirm") -> ()  [unwired: 1 out]
              }
            }
            n85 = for {
              tunnel: w194 -> [w216] mode=indexing
              tunnel: w193 -> [w218] mode=indexing
              tunnel: w192 -> [w219]
              tunnel: w191 -> [w217] mode=indexing
              tunnel: [w215] -> w190 mode=indexing
              n86 = Bundle By Name(cluster=w219, "x(mm)"=w218, "y(mm)"=w217, "z(mm)"=w216) -> (w215:cluster{"x(mm)":dbl, "y(mm)":dbl, "z(mm)":dbl})
            }
            n87 = Bundle By Name(cluster=w212, "FollowScan"=w190, "3DProfileToPlot"=w190, "FollowScanZOffset(mm)"="Follow Z offset(mm)", "ProbeRadius(mm)"="Probe Radius(2mm)") -> (w213:T15)
            n88 = property on="Interpolate Scan" class="Bool"(error in=w198, "DisabledEnum"=T6."Enabled" ("Disabled")) -> (error out=w205:errorcluster)  [unwired: 1 in, 1 out]
            n89 = call <vilib>:"Add State(s) to Queue__JKI_lib_State_Machine.vi"("State(s) in Front (\"\")"="LJT4: RestEncoder\nUtility: Plot3D" ("State(s) in Front (\"\")"), "State(s) in (\"\")"=w202) -> ("States Out"=w203:string)  [unwired: 13 in]
          }
          event "Remove Z outlier": Value Change {
            n90 = event-data() -> ()  [unwired: 1 in, 6 out]
            n91 = Unbundle By Name(w246) -> ("Raw3DProfile"=w247:cluster{"x(mm)":dbl, "y(mm)":dbl, "z(mm)":dbl}[])
            n92 = for {
              tunnel: w247 -> [w250] mode=indexing
              tunnel: "Upper Z limite(mm)" -> [w253]
              shift-right: [w251] -> w237
              shift-left: cluster{"x(mm)":dbl, "y(mm)":dbl, "z(mm)":dbl}[] [] -> [w249]
              n93 = Unbundle By Name(w250) -> ("z(mm)"=w254:dbl)
              n94 = Less Or Equal?(x=w254, y=w253) -> (x <= y?=w252:bool)
              n95 = case shown="True" w252 {
                tunnel: [w255 w258] -> w251
                tunnel: w250 -> [_ w257]
                tunnel: w249 -> [w255 w256]
                frame False {
                }
                frame True {
                  n96 = Build Array (concatenate)(w256, w257) -> (w258:cluster{"x(mm)":dbl, "y(mm)":dbl, "z(mm)":dbl}[])
                }
              }
            }
            n97 = property on="Calc follow scan" class="Bool"(error in=w238, "DisabledEnum"=T6."Enabled" ("Disabled")) -> (error out=w239:errorcluster)  [unwired: 1 in, 1 out]
            n98 = Bundle By Name(cluster=w246, "3DProfile"=w237, "3DProfileToPlot"=w237) -> (w245:T15)
            n99 = call <vilib>:"Add State(s) to Queue__JKI_lib_State_Machine.vi"("State(s) in Front (\"\")"="Utility: Plot3D" ("State(s) in Front (\"\")"), "State(s) in (\"\")"=w244) -> ("States Out"=w243:string)  [unwired: 13 in]
          }
          event "Interpolate Scan": Value Change {
            n100 = event-data() -> ()  [unwired: 1 in, 6 out]
            n101 = Unbundle By Name(w272) -> ("FollowScan"=w274:cluster{"x(mm)":dbl, "y(mm)":dbl, "z(mm)":dbl}[])
            n102 = call "InterpRoute.vi"("error in (no error)"=w260, "GridSize(mm)"="FollowScanGridSize(mm)", "FollowScanWOffset"=w274) -> ("error out"=w259:errorcluster, "Zi"=w262:dbl[], "Yi"=w269:dbl[], "Xi"=w270:dbl[])  [unwired: 4 in, 1 out]
            n103 = Index Array(array=w274) -> (element=w273:cluster{"x(mm)":dbl, "y(mm)":dbl, "z(mm)":dbl})  [unwired: 1 in]
            n104 = property on="Follow Scan" class="Bool"(error in=w259, "DisabledEnum"=T6."Enabled" ("Disabled")) -> (error out=w267:errorcluster)  [unwired: 1 in, 1 out]
            n105 = for {
              tunnel: w273 -> [w279]
              tunnel: w270 -> [w278] mode=indexing
              tunnel: w269 -> [w277] mode=indexing
              tunnel: w262 -> [w276] mode=indexing
              tunnel: [w275] -> w263 mode=indexing
              n106 = Bundle By Name(cluster=w279, "x(mm)"=w278, "y(mm)"=w277, "z(mm)"=w276) -> (w275:cluster{"x(mm)":dbl, "y(mm)":dbl, "z(mm)":dbl})
            }
            n107 = Bundle By Name(cluster=w272, "FollowScanWInter"=w263, "3DProfileToPlot"=w263, "FollowGridSize(mm)"="FollowScanGridSize(mm)") -> (w271:T15)
            n108 = call <vilib>:"Add State(s) to Queue__JKI_lib_State_Machine.vi"("State(s) in Front (\"\")"="Utility: Plot3D" ("State(s) in Front (\"\")"), "State(s) in (\"\")"=w265) -> ("States Out"=w264:string)  [unwired: 13 in]
          }
          event "Follow Scan": Value Change {
            w286 = TRUE ("event data")
            w298 = "\r"
            # "set feedrate"
            n109 = event-data() -> ()  [unwired: 1 in, 6 out]
            n110 = call "RemoteEventFGV.vi"() -> ("Remote Event out"=w284:T16)  [unwired: 10 in, 1 out]
            n111 = Unbundle By Name(w284) -> ("remote start event"=w283:refnum<user-event>)
            n112 = Unbundle By Name(w311) -> ("FollowScanWInter"=w293:cluster{"x(mm)":dbl, "y(mm)":dbl, "z(mm)":dbl}[])
            n113 = Generate User Event(priority (normal)=usereventprio."high priority", user event=w283, event data cluster=TRUE ("event data")) -> (error out=w280:errorcluster)  [unwired: 1 in, 1 out]
            n114 = Number To Fractional String(number="Follow Speed (mm/min)", precision (6)=i16 3) -> (F-format string=w307:string)  [unwired: 2 in]
            n115 = Concatenate Strings("F" ("string"), w307, "\r") -> (w306:string)
            n116 = call "Send-Receive Serial Port.vi"("Data to write"=w306, "error in (no error)"=w289) -> ("error out"=w303:errorcluster)  [unwired: 12 in, 1 out]
            n117 = Concatenate Strings("$120=200" ("string"), w298) -> (w297:string)
            n118 = Concatenate Strings("$121=200" ("string"), w298) -> (w296:string)
            n119 = Concatenate Strings("$122=200" ("string"), w298) -> (w295:string)
            n120 = local write "FollowScan"(w286) -> ()
            n121 = Generate User Event(user event=w290, event data cluster=w286, error in=w289) -> (error out=w285:errorcluster)  [unwired: 1 in, 1 out]
            n122 = Build Array(w297, w296, w295) -> (w294:string[])
            n123 = for {
              shift-right: [w313] -> w302
              shift-left: w303 -> [w314]
              tunnel: w294 -> [w312] mode=indexing
              n124 = call "Send-Receive Serial Port.vi"("Data to write"=w312, "error in (no error)"=w314) -> ("error out"=w313:errorcluster)  [unwired: 12 in, 1 out]
            }
            n125 = Generate User Event(user event=w310, event data cluster=w293, error in=w302) -> (error out=w288:errorcluster)  [unwired: 1 in, 1 out]
            n126 = call <vilib>:"Add State(s) to Queue__JKI_lib_State_Machine.vi"("State(s) in (\"\")"=w291) -> ("States Out"=w292:string)  [unwired: 14 in]
            n127 = Merge Errors(w288, w285, w280) -> (w287:errorcluster)
          }
          event "ShowFLImIntensity": Value Change {
            n128 = event-data() -> ()  [unwired: 1 in, 6 out]
            n129 = Obtain Queue(name (unnamed)="LocationData", element data type=cluster{"Time":dbl, "x":dbl} {"Time"=0.0, "x"=0.0}, error in (no error)=w331) -> (queue out=w332:refnum<queue>, error out=w333:errorcluster)  [unwired: 2 in, 1 out]
            n130 = Unbundle By Name(w320) -> ("ScanOrigin"=w325:cluster{"X":sgl, "Y":sgl, "Z":sgl}, "BG(V)"=w324:dbl, "YPixelSize(mm)"=w322:dbl)
            n131 = Flush Queue(queue=w332, error in (no error)=w333) -> (remaining elements=w319:cluster{"Time":dbl, "x":dbl}[], error out=w329:errorcluster)  [unwired: 1 out]
            n132 = for {
              tunnel: w319 -> [w339] mode=indexing
              tunnel: [w337] -> w326 mode=indexing
              n133 = Unbundle By Name(w339) -> ("x"=w336:dbl, "Time"=w335:dbl)
              n134 = Bundle("x"=w336, 0.0, "Time"=w335) -> (w337:cluster{"x":dbl, dbl, "Time":dbl})  [unwired: 1 in]
            }
            n135 = local write "Tab Control"(T2."IntensityGraph" ("Tab Control")) -> ()
            n136 = call "GetPPIXImg.vi"("Background"=w324, "dy"=w322, "Origin"=w325, "3D Profile in"=w326) -> ("Z"=w316:dbl[], "Y"=w317:dbl[], "X"=w318:dbl[])  [unwired: 4 in, 1 out]
            n137 = Bundle("X"=w318, "Y"=w317, "Z"=w316) -> (w315:cluster{"X":dbl[], "Y":dbl[], "Z":dbl[]})  [unwired: 1 in]
            n138 = call-poly <vilib>:"Plot Helper.vi"("z vector"=w316, "y vector"=w317, "x vector"=w318) -> ("3D Plot lvclass Array out"=→"CH1":refnum<class "3D Plot Datatype.lvclass">[])  [unwired: 3 in, 5 out]
            n139 = Bundle By Name(cluster=w320, "RawFollowScanData"=w319, "PPIXProcessedImg"=w315) -> (w321:T15)
          }
          event "Home": Value Change {
            n140 = event-data() -> ()  [unwired: 1 in, 6 out]
            n141 = call <vilib>:"Add State(s) to Queue__JKI_lib_State_Machine.vi"("State(s) in Front (\"\")"="Stage: Home" ("State(s) in Front (\"\")"), "State(s) in (\"\")"=w342) -> ("States Out"=w343:string)  [unwired: 13 in]
          }
          event "Hault": Value Change {
            n142 = event-data() -> ()  [unwired: 1 in, 6 out]
            n143 = call <vilib>:"Add State(s) to Queue__JKI_lib_State_Machine.vi"("State(s) in Front (\"\")"="Stage: Reset" ("State(s) in Front (\"\")"), "State(s) in (\"\")"=w348) -> ("States Out"=w347:string)  [unwired: 13 in]
          }
          event "X++": Value Change {
            n144 = event-data() -> ()  [unwired: 1 in, 6 out]
            n145 = Unbundle By Name(w360) -> ("StepSize"=w353:dbl)
            n146 = call "Get Status.vi"("error in (no error)"=w350) -> ("Status"=w357:T9, "Current position"=w354:cluster{"X":sgl, "Y":sgl, "Z":sgl}, "error out"=w352:errorcluster)  [unwired: 10 in, 2 out]
            n147 = Equal?(x=Status."Idle" ("Status"), y=w357) -> (x = y?=w355:bool)
            n148 = case shown="True" w355 {
              tunnel: w354 -> [_ w370]
              tunnel: w353 -> [_ w363]
              tunnel: w352 -> [w362 w366]
              tunnel: [w362 w365] -> w351
              frame False {
                n149 = One Button Dialog(message="Stage is not Idle!\nPlease try again when stage is Idle. ") -> ()  [unwired: 1 in, 1 out]
              }
              frame True {
                n150 = Unbundle By Name(w370) -> ("X"=w364:sgl, "Y"=w368:sgl, "Z"=w367:sgl)
                n151 = Add(x=w364, y=w363) -> (x+y=w369:dbl)
                n152 = call "Go to Position.vi"("X (mm)"=w369, "Y (mm)"=w368, "Z (mm)"=w367, "error in (no error)"=w366) -> ("error out"=w365:errorcluster)  [unwired: 11 in]
              }
            }
            n153 = call <vilib>:"Add State(s) to Queue__JKI_lib_State_Machine.vi"("State(s) in (\"\")"=w358) -> ("States Out"=w359:string)  [unwired: 14 in]
          }
          event "Y++": Value Change {
            n154 = event-data() -> ()  [unwired: 1 in, 6 out]
            n155 = Unbundle By Name(w381) -> ("StepSize"=w374:dbl)
            n156 = call "Get Status.vi"("error in (no error)"=w371) -> ("Status"=w378:T9, "Current position"=w375:cluster{"X":sgl, "Y":sgl, "Z":sgl}, "error out"=w373:errorcluster)  [unwired: 10 in, 2 out]
            n157 = Equal?(x=Status."Idle" ("Status"), y=w378) -> (x = y?=w376:bool)
            n158 = case shown="True" w376 {
              tunnel: w375 -> [_ w391]
              tunnel: w374 -> [_ w387]
              tunnel: w373 -> [w383 w389]
              tunnel: [w383 w388] -> w372
              frame False {
                n159 = One Button Dialog(message="Stage is not Idle!\nPlease try again when stage is Idle. ") -> ()  [unwired: 1 in, 1 out]
              }
              frame True {
                n160 = Unbundle By Name(w391) -> ("X"=w384:sgl, "Y"=w386:sgl, "Z"=w390:sgl)
                n161 = Add(x=w386, y=w387) -> (x+y=w385:dbl)
                n162 = call "Go to Position.vi"("X (mm)"=w384, "Y (mm)"=w385, "Z (mm)"=w390, "error in (no error)"=w389) -> ("error out"=w388:errorcluster)  [unwired: 11 in]
              }
            }
            n163 = call <vilib>:"Add State(s) to Queue__JKI_lib_State_Machine.vi"("State(s) in (\"\")"=w379) -> ("States Out"=w380:string)  [unwired: 14 in]
          }
          event "GoToZero": Value Change {
            n164 = event-data() -> ()  [unwired: 1 in, 6 out]
            n165 = call <vilib>:"Add State(s) to Queue__JKI_lib_State_Machine.vi"("State(s) in Front (\"\")"="Stage: GoToZero" ("State(s) in Front (\"\")"), "State(s) in (\"\")"=w393) -> ("States Out"=w394:string)  [unwired: 13 in]
          }
          event "Y--": Value Change {
            n166 = event-data() -> ()  [unwired: 1 in, 6 out]
            n167 = Unbundle By Name(w407) -> ("StepSize"=w400:dbl)
            n168 = call "Get Status.vi"("error in (no error)"=w397) -> ("Status"=w404:T9, "Current position"=w401:cluster{"X":sgl, "Y":sgl, "Z":sgl}, "error out"=w399:errorcluster)  [unwired: 10 in, 2 out]
            n169 = Equal?(x=Status."Idle" ("Status"), y=w404) -> (x = y?=w402:bool)
            n170 = case shown="True" w402 {
              tunnel: w401 -> [_ w417]
              tunnel: w400 -> [_ w413]
              tunnel: w399 -> [w409 w415]
              tunnel: [w409 w414] -> w398
              frame False {
                n171 = One Button Dialog(message="Stage is not Idle!\nPlease try again when stage is Idle. ") -> ()  [unwired: 1 in, 1 out]
              }
              frame True {
                n172 = Unbundle By Name(w417) -> ("X"=w410:sgl, "Y"=w412:sgl, "Z"=w416:sgl)
                n173 = Subtract(x=w412, y=w413) -> (x-y=w411:dbl)
                n174 = call "Go to Position.vi"("X (mm)"=w410, "Y (mm)"=w411, "Z (mm)"=w416, "error in (no error)"=w415) -> ("error out"=w414:errorcluster)  [unwired: 11 in]
              }
            }
            n175 = call <vilib>:"Add State(s) to Queue__JKI_lib_State_Machine.vi"("State(s) in (\"\")"=w405) -> ("States Out"=w406:string)  [unwired: 14 in]
          }
          event "Z--": Value Change {
            n176 = event-data() -> ()  [unwired: 1 in, 6 out]
            n177 = Unbundle By Name(w428) -> ("StepSize"=w421:dbl)
            n178 = call "Get Status.vi"("error in (no error)"=w418) -> ("Status"=w425:T9, "Current position"=w422:cluster{"X":sgl, "Y":sgl, "Z":sgl}, "error out"=w420:errorcluster)  [unwired: 10 in, 2 out]
            n179 = Equal?(x=Status."Idle" ("Status"), y=w425) -> (x = y?=w423:bool)
            n180 = case shown="True" w423 {
              tunnel: w422 -> [_ w438]
              tunnel: w421 -> [_ w435]
              tunnel: w420 -> [w430 w437]
              tunnel: [w430 w436] -> w419
              frame False {
                n181 = One Button Dialog(message="Stage is not Idle!\nPlease try again when stage is Idle. ") -> ()  [unwired: 1 in, 1 out]
              }
              frame True {
                n182 = Unbundle By Name(w438) -> ("X"=w434:sgl, "Y"=w433:sgl, "Z"=w431:sgl)
                n183 = Subtract(x=w431, y=w435) -> (x-y=w432:dbl)
                n184 = call "Go to Position.vi"("X (mm)"=w434, "Y (mm)"=w433, "Z (mm)"=w432, "error in (no error)"=w437) -> ("error out"=w436:errorcluster)  [unwired: 11 in]
              }
            }
            n185 = call <vilib>:"Add State(s) to Queue__JKI_lib_State_Machine.vi"("State(s) in (\"\")"=w426) -> ("States Out"=w427:string)  [unwired: 14 in]
          }
          event "Z++": Value Change {
            n186 = event-data() -> ()  [unwired: 1 in, 6 out]
            n187 = Unbundle By Name(w449) -> ("StepSize"=w442:dbl)
            n188 = call "Get Status.vi"("error in (no error)"=w439) -> ("Status"=w446:T9, "Current position"=w443:cluster{"X":sgl, "Y":sgl, "Z":sgl}, "error out"=w441:errorcluster)  [unwired: 10 in, 2 out]
            n189 = Equal?(x=Status."Idle" ("Status"), y=w446) -> (x = y?=w444:bool)
            n190 = case shown="True" w444 {
              tunnel: w443 -> [_ w459]
              tunnel: w442 -> [_ w456]
              tunnel: w441 -> [w451 w458]
              tunnel: [w451 w457] -> w440
              frame False {
                n191 = One Button Dialog(message="Stage is not Idle!\nPlease try again when stage is Idle. ") -> ()  [unwired: 1 in, 1 out]
              }
              frame True {
                n192 = Unbundle By Name(w459) -> ("X"=w455:sgl, "Y"=w454:sgl, "Z"=w452:sgl)
                n193 = Add(x=w452, y=w456) -> (x+y=w453:dbl)
                n194 = call "Go to Position.vi"("X (mm)"=w455, "Y (mm)"=w454, "Z (mm)"=w453, "error in (no error)"=w458) -> ("error out"=w457:errorcluster)  [unwired: 11 in]
              }
            }
            n195 = call <vilib>:"Add State(s) to Queue__JKI_lib_State_Machine.vi"("State(s) in (\"\")"=w447) -> ("States Out"=w448:string)  [unwired: 14 in]
          }
          event "Set Origin": Value Change {
            # "reset encoder"
            n196 = event-data() -> ()  [unwired: 1 in, 6 out]
            n197 = call "Get Status.vi"("error in (no error)"=w465) -> ("Current position"=w468:cluster{"X":sgl, "Y":sgl, "Z":sgl}, "error out"=w461:errorcluster)  [unwired: 10 in, 3 out]
            "Scan Origin MPos" <- w468
            n198 = call "LabJack_FGV_T4.vi"("Operation(Read)"=enum16{"Write", "Read"}."Read" ("Operation"), "error in (no error)"=w461) -> ("error out"=w464:errorcluster, "Read data"=w463:i32)  [unwired: 8 in]
            n199 = Bundle By Name(cluster=w470, "ScanOrigin"=w468) -> (w469:T15)
            n200 = call "LJM_eReadName.vi"("Handle In"=w463, "Name"="DIO4_EF_READ_A_AND_RESET", "error in"=w464) -> ("error out"=w460:errorcluster)  [unwired: 10 in, 2 out]
          }
          event "3DProfileScan": Value Change {
            # "set feedrate"
            # "Flush queue"
            n201 = event-data() -> ()  [unwired: 1 in, 6 out]
            n202 = Unbundle By Name(w478) -> ("ScanOrigin"=w491:cluster{"X":sgl, "Y":sgl, "Z":sgl})
            n203 = Flush Queue(queue=w488, error in (no error)=w487) -> (error out=w486:errorcluster)  [unwired: 2 out]
            n204 = call "RoutePlaner.vi"("Origin In"=w491, "Pixel Size(mm)"="Y Pixel Size(mm)", "Y distance(mm)"="Y distance(mm)", "X distance (mm)"="X distance (mm)") -> ("PtArray"=w475:cluster{"x":dbl, "y":dbl, "z":dbl}[])  [unwired: 6 in, 1 out]
            n205 = Number To Fractional String(number="Pre Scan Speed (mm/min)", precision (6)=i16 3) -> (F-format string=w482:string)  [unwired: 2 in]
            n206 = Concatenate Strings("F" ("string"), w482, "\r") -> (w481:string)
            n207 = call "Send-Receive Serial Port.vi"("Data to write"=w481, "error in (no error)"=w486) -> ("error out"=w474:errorcluster)  [unwired: 12 in, 1 out]
            n208 = Generate User Event(user event=w476, event data cluster=w475, error in=w474) -> (error out=w473:errorcluster)  [unwired: 1 in, 1 out]
            n209 = Bundle By Name(cluster=w478, "YPixelSize(mm)"="Y Pixel Size(mm)") -> (w479:T15)
            n210 = call <vilib>:"Set Busy.vi"("error in (no error)"=w473) -> ("error out"=w471:errorcluster)  [unwired: 9 in, 1 out]
            n211 = call <vilib>:"Add State(s) to Queue__JKI_lib_State_Machine.vi"("State(s) in Front (\"\")"="AccuRange: Start" ("State(s) in Front (\"\")"), "State(s) in (\"\")"=w490) -> ("States Out"=w489:string)  [unwired: 13 in]
          }
          event "X--": Value Change {
            n212 = event-data() -> ()  [unwired: 1 in, 6 out]
            n213 = Unbundle By Name(w504) -> ("StepSize"=w497:dbl)
            n214 = call "Get Status.vi"("error in (no error)"=w494) -> ("Status"=w501:T9, "Current position"=w498:cluster{"X":sgl, "Y":sgl, "Z":sgl}, "error out"=w496:errorcluster)  [unwired: 10 in, 2 out]
            n215 = Equal?(x=Status."Idle" ("Status"), y=w501) -> (x = y?=w499:bool)
            n216 = case shown="True" w499 {
              tunnel: w498 -> [_ w514]
              tunnel: w497 -> [_ w508]
              tunnel: w496 -> [w506 w510]
              tunnel: [w506 w509] -> w495
              frame False {
                n217 = One Button Dialog(message="Stage is not Idle!\nPlease try again when stage is Idle. ") -> ()  [unwired: 1 in, 1 out]
              }
              frame True {
                n218 = Unbundle By Name(w514) -> ("X"=w507:sgl, "Y"=w512:sgl, "Z"=w511:sgl)
                n219 = Subtract(x=w507, y=w508) -> (x-y=w513:dbl)
                n220 = call "Go to Position.vi"("X (mm)"=w513, "Y (mm)"=w512, "Z (mm)"=w511, "error in (no error)"=w510) -> ("error out"=w509:errorcluster)  [unwired: 11 in]
              }
            }
            n221 = call <vilib>:"Add State(s) to Queue__JKI_lib_State_Machine.vi"("State(s) in (\"\")"=w502) -> ("States Out"=w503:string)  [unwired: 14 in]
          }
          event "Jog Step Size(mm)": Value Change {
            n222 = event-data() -> ("NewVal"=w516:dbl)  [unwired: 1 in, 5 out]
            n223 = Bundle By Name(cluster=w519, "StepSize"=w516) -> (w518:T15)
          }
          event "Quit": Value Change {
            # "Exit Button Value Change (pressed) Event\n(this executes Macro: Exit to terminate the VI)"
            n224 = event-data() -> ()  [unwired: 1 in, 1 out]
            n225 = call <vilib>:"Add State(s) to Queue__JKI_lib_State_Machine.vi"("State(s) in Front (\"\")"="Macro: Exit", "State(s) in (\"\")"=w524) -> ("States Out"=w523:string)  [unwired: 13 in]
          }
          event "Start": Value Change {
            n226 = event-data() -> ()  [unwired: 1 in, 6 out]
            n227 = call <vilib>:"Add State(s) to Queue__JKI_lib_State_Machine.vi"("State(s) in Front (\"\")"="AccuRange: Start" ("State(s) in Front (\"\")"), "State(s) in (\"\")"=w528) -> ("States Out"=w527:string)  [unwired: 13 in]
          }
          event "Stop": Value Change {
            n228 = event-data() -> ()  [unwired: 1 in, 6 out]
            n229 = call <vilib>:"Add State(s) to Queue__JKI_lib_State_Machine.vi"("State(s) in Front (\"\")"="AccuRange: Stop" ("State(s) in Front (\"\")"), "State(s) in (\"\")"=w533) -> ("States Out"=w532:string)  [unwired: 13 in]
          }
          event Panel Close? {
            # "Discard the event because we'll close the front panel ourselves in Macro: Exit"
            # "Close Panel button (pressed) Event\n(this executes Macro: Exit to terminate the VI)"
            n230 = event-data() -> ()  [unwired: 1 in, 1 out]
            n231 = call <vilib>:"Add State(s) to Queue__JKI_lib_State_Machine.vi"("State(s) in Front (\"\")"="Macro: Exit", "State(s) in (\"\")"=w540) -> ("States Out"=w539:string)  [unwired: 13 in]
            n232 = event-data("Discard?"=TRUE) -> ()  [unwired: 1 in, 1 out]
          }
        }
      }
      frame "---------- Macro ----------" {
        # "Do not put any code in this frame.\n(It is a separator no-op. You can make a copy of this frame to create a new Macro frame)"
        n233 = call <vilib>:"Add State(s) to Queue__JKI_lib_State_Machine.vi"("State(s) in (\"\")"=w545) -> ("States Out"=w544:string)  [unwired: 14 in]
      }
      frame "Macro: SaveData" {
        # "Save 3D profile and scan data\n()"
        n234 = call <vilib>:"Add State(s) to Queue__JKI_lib_State_Machine.vi"("State(s) in Front (\"\")"="Data: OpenTDMS\nData: SaveExpDetail\nData: SaveRaw3DProfile\nData: SaveProcessed3DProfile\nData: SaveFollowScan\nData: SaveInterpedFollowScan\nData: SaveRawFollowScanData\nData: SaveProcessedPPIXImg\nData: CloseTDMS\nDialog: DataSaved" ("State(s) in Front (\"\")"), "State(s) in (\"\")"=w551) -> ("States Out"=w550:string)  [unwired: 13 in]
      }
      frame "Macro: Initialize" {
        # "Initialization Macro\n(This is called once, when the VI starts)"
        n235 = call <vilib>:"Add State(s) to Queue__JKI_lib_State_Machine.vi"("State(s) in Front (\"\")"="Data: Initialize\nInitialize Core Data\nUI: Initialize\nUI: Front Panel State >> Open\nData: UpdateStepSize\nUI: StartUp\nUI: Cursor Set >> Busy\nStage: Initialize\nUI: Update\nAccuRange: Initialize\nUI: Update\nLJT4: Initialize\nUI: Update\n/*USBCam: Initialize\nLJT4: Config\nStage: Reset\nStage: Config\nAccuRange: Config\nAccuRange: Start\nData: CreatDataFolder\nUI: Cursor Set >> Idle\nStage: Home\nStage: GoToZero\nUI: Update", "State(s) in (\"\")"=w552) -> ("States Out"=w557:string)  [unwired: 13 in]
      }
      frame "Macro: Exit" {
        # "Exit Macro\n(This is called once, when the VI exits)"
        n236 = Unbundle By Name(w566) -> ("Core.Close Panel on Exit?"=w565:bool)
        n237 = Select(t="UI: Front Panel State >> Close", s=w565, f="") -> (s? t:f=w562:string)
        n238 = call <vilib>:"Add State(s) to Queue__JKI_lib_State_Machine.vi"("State(s) in Front (\"\")"="AccuRange: Stop\nStage: Close\nAccuRange: Close\nLJT4: Close\n/*USBCam: Close\nUI: Update\nUtility: DestroyQueue" ("State(s) in Front (\"\")"), "State(s) in (\"\")"=w562, "State(s) at Back (\"\")"="Data: Cleanup\nExit") -> ("States Out"=w560:string)  [unwired: 12 in]
        n239 = call <vilib>:"Add State(s) to Queue__JKI_lib_State_Machine.vi"("State(s) in Front (\"\")"=w560, "State(s) in (\"\")"=w569) -> ("States Out"=w568:string)  [unwired: 13 in]
      }
      frame "---------- Core ----------" {
        # "Do not put any code in this frame.\n(it is a separator no-op)"
        n240 = call <vilib>:"Add State(s) to Queue__JKI_lib_State_Machine.vi"("State(s) in (\"\")"=w574) -> ("States Out"=w573:string)  [unwired: 14 in]
      }
      frame Default {
        w585 = 42 items=["No error", "Argument error", "Memory is full", "Out of zone", "End of file", "File already open", "Generic file I/O error", "File not found", "File permission error", "Disk is full", "Duplicate path", "Too many files open", "System feature not enabled", "Resource file not found", "Cannot add resource", "Resource not found", "Image not found", "Image memory error", "Pen does not exist", "Config type invalid", "Config token not found", "Config parse error", "Config memory error", "Bad external code format", "Bad external code offset", "External code not present", "Null window", "Destroy window error", "Null menu", "Print aborted", "Bad print record", "Print driver error", "Windows error during printing", "Memory error during printing", "Print dialog error", "Generic print error", "Invalid device refnum", "Device not found", "Device parameter error", "Device unit error", "Cannot open device", "Device call aborted", "Generic error", "Cancelled by user", "Object ID too low", "Object ID too high", "Object not in heap", "Unknown heap", "Unknown object (invalid DefProc)", "Unknown object (DefProc not in table)", "Message out of range", "Invalid (null) method", "Unknown message", "Manager call not supported", "Bad address", "Network operation in progress", "Network operation timed out", "Connection is busy", "Network attribute not supported", "Network error", "Address in use", "System out of memory", "Connection aborted", "Connection refused", "Not connected", "Already connected", "Connection closed", "Initialization error (interapplication manager)", "Bad occurrence", "Wait on unbound occurrence handler", "Occurrence queue overflow", "Datalog type conflict", "Unused", "Unrecognized type (interapplication manager)", "Memory corrupt", "Failed to make temporary DLL", "Old CIN version", "Drag socket not found", "Failed to load drop-object", "Failed to register OLE object", "Failed to release OLE object", "Format specifier type mismatch", "Unknown format specifier", "Too few format specifiers", "Too many format specifiers", "Scan failed", "Newer CIN version", "Error converting to variant", "Runtime menu error", "Password tampered", "Variant attribute not found", "Incompatible variant data type", "Event data is not available", "Event Store is not present", "Occurrence is not found", "Event Queue is not created", "Event info is not available", "Refnum passed is NULL", "Error retrieving Class GUID", "Error retrieving CoClass GUID", "Error retrieving TypeLib GUID.", "Bad built application magic bytes.", "Specific driver is different from the specific driver associated with the Logical Name.", "There is no session opened to the class driver.", "Max Error", "MAX - Error with config objects", "MAX - Error loading configuration", "MAX - Group not supported"]
        # "Current State"
        # "Do not delete, rename, or modify this frame.\n(this is used to capture unhandled states and typos)"
        # "Handle mistyped state name (developer tool)"
        n241 = Format Into String(format string="Software Exception: Unhandled State \"%s\"." ("message"), error in=w581, w576) -> (resulting string=w584:string, error out=w583:errorcluster)  [unwired: 1 in]
        n242 = call <vilib>:"Error Cluster From Error Code.vi"("show call chain? (False)"=TRUE, "error in (no error)"=w583, "error message (\"\")"=w584, "error code (0)"=w585) -> ("error out"=w582:errorcluster)  [unwired: 5 in]
        n243 = call <vilib>:"Add State(s) to Queue__JKI_lib_State_Machine.vi"("State(s) in (\"\")"=w580) -> ("States Out"=w579:string)  [unwired: 14 in]
      }
      frame "Initialize Core Data" {
        # "Do not delete, rename, or modify this frame.\n(this is used to determine panel behavior on exit)"
        # "originally closed?"
        # "exe?"
        # "If panel starts closed or is an EXE, then close it when we exit"
        n244 = property class="VI"() -> ("FP.State"=w590:T10)  [unwired: 2 in, 2 out]
        n245 = property class="App"() -> ("App.Kind"=w596:T11)  [unwired: 2 in, 2 out]
        n246 = control-ref of="Current VI Reference"() -> (w591:refnum<vi>)
        n247 = Equal?(x=w590, y=T10."Closed" ("Front Panel Window:State")) -> (x = y?=w588:bool)
        n248 = Equal?(x=w596, y=T11."Run Time System" ("Application:Kind")) -> (x = y?=w594:bool)
        n249 = Or(x=w588, y=w594) -> (x .or. y?=w592:bool)
        n250 = Bundle By Name(cluster=w593, "Core.Current VI Reference"=w591, "Core.Close Panel on Exit?"=w592) -> (w598:T15)
        n251 = call <vilib>:"Add State(s) to Queue__JKI_lib_State_Machine.vi"("State(s) in (\"\")"=w600) -> ("States Out"=w599:string)  [unwired: 14 in]
      }
      frame "Error Handler" {
        # "Unhandled Error -- Display it"
        # "Handle any errors here.\nYou can also output any states to clean-up after errors occur"
        # "Clear error"
        n252 = call <vilib>:"General Error Handler.vi"("error in (no error)"=w603) -> ()  [unwired: 10 in, 5 out]
        n253 = call <vilib>:"Add State(s) to Queue__JKI_lib_State_Machine.vi"("State(s) in Front (\"\")"="/* Post Error States\nMacro: Exit", "State(s) in (\"\")"=w607) -> ("States Out"=w606:string)  [unwired: 13 in]
      }
      frame "Exit" {
        # "Do not put any code in this frame.\n(No errors that occur here will be handled.)"
        n254 = Generate User Event(user event=w611, event data cluster=TRUE ("event data"), error in=w609) -> (error out=w610:errorcluster)  [unwired: 1 in, 1 out]
        n255 = call <vilib>:"Add State(s) to Queue__JKI_lib_State_Machine.vi"("State(s) in (\"\")"=w616) -> ("States Out"=w615:string)  [unwired: 14 in]
      }
      frame "---------- Data ----------" {
        # "Do not put any code in this frame.\n(It is a separator no-op. You can make a copy of this frame to create a new Data frame)"
        n256 = call <vilib>:"Add State(s) to Queue__JKI_lib_State_Machine.vi"("State(s) in (\"\")"=w621) -> ("States Out"=w620:string)  [unwired: 14 in]
      }
      frame "Data: Initialize" {
        w622 = 0.0  # FollowGridSize(mm)
        w623 = 0.0  # ProbeRadius(mm)
        w624 = cluster{"x":dbl[], "y":dbl[], "Time(ms)":dbl[]} {"x"=[], "y"=[], "Time(ms)"=[]}  # PPIXProcessedImg
        w625 = cluster{"Time(ms)":dbl, "x":dbl}[] []  # RawFollowScanData
        w626 = 0.0  # FollowScanZOffset(mm)
        w627 = cluster{"x":dbl, "y":dbl} {"x"=-21.5, "y"=-70.0}  # FiberOffset
        w628 = refnum<k34> refnum  # tdms file
        w629 = cluster{"x(mm)":dbl, "y(mm)":dbl, "z(mm)":dbl}[] []  # Raw3DProfileNoY
        w630 = path ""  # SaveFilePath
        w631 = cluster{"x(mm)":dbl, "y(mm)":dbl, "z(mm)":dbl}[] []  # FollowScan
        w632 = cluster{"x(mm)":dbl, "y(mm)":dbl, "z(mm)":dbl}[] []  # 3DProfileToPlot
        w635 = cluster{"X":sgl, "Y":sgl, "Z":sgl} {"X"=0.0, "Y"=0.0, "Z"=0.0}  # HomeMposOrigin
        w636 = FALSE  # StageHomed?
        w637 = 0.0  # BG(V)
        w638 = cluster{"x(mm)":dbl, "y(mm)":dbl, "z(mm)":dbl}[] []  # FollowScanWInter
        w639 = 0.0  # YPixelSize(mm)
        w640 = cluster{"x(mm)":dbl, "y(mm)":dbl, "z(mm)":dbl}[] []  # Raw3DProfile
        w641 = cluster{"x(mm)":dbl, "y(mm)":dbl, "z(mm)":dbl}[] []  # 3DProfile
        w642 = T4 refnum  # USBCam
        w643 = T5 refnum  # IMAQ
        w644 = 0  # Tic
        w645 = cluster{"X":sgl, "Y":sgl, "Z":sgl} {"X"=0.0, "Y"=0.0, "Z"=0.0}  # ScanOrigin
        w646 = 5.0  # StepSize
        w647 = refnum<visa-resource-name> "COM5"  # RangeCOM
        w648 = refnum<visa-resource-name> "COM3"  # StageCOM
        w634 = T1 {"Stage"=FALSE, "T4"=FALSE, "RangerFinder"=FALSE, "USB Cam"=FALSE}  # Sys Status
        w649 = T17 {"Current VI Reference"=refnum, "Close Panel on Exit?"=FALSE}  # Core
        # "Initialize the shift-register data, here.\n(data names are defined by what you wire into the bundle function)"
        n257 = Bundle("Core"=w649, "Sys Status"=w634, "StageCOM"=w648, "RangeCOM"=w647, "StepSize"=w646, "ScanOrigin"=w645, "HomeMposOrigin"=w635, "Tic"=w644, "IMAQ"=w643, "USBCam"=w642, "3DProfile"=w641, "Raw3DProfile"=w640, "FollowScanZOffset(mm)"=w626, "YPixelSize(mm)"=w639, "FollowScanWInter"=w638, "BG(V)"=w637, "StageHomed?"=w636, "3DProfileToPlot"=w632, "FollowScan"=w631, "SaveFilePath"=w630, "Raw3DProfileNoY"=w629, "tdms file"=w628, "FiberOffset"=w627, "RawFollowScanData"=w625, "PPIXProcessedImg"=w624, "ProbeRadius(mm)"=w623, "FollowGridSize(mm)"=w622) -> (w651:T15)  [unwired: 1 in]
        n258 = call <vilib>:"Add State(s) to Queue__JKI_lib_State_Machine.vi"("State(s) in (\"\")"=w653) -> ("States Out"=w652:string)  [unwired: 14 in]
      }
      frame "Data: UpdateStepSize" {
        # "Template Separator\n(You can make a copy of, or modify, this frame)"
        n259 = Bundle By Name(cluster=w656, "StepSize"="Jog Step Size(mm)") -> (w657:T15)
        n260 = call <vilib>:"Add State(s) to Queue__JKI_lib_State_Machine.vi"("State(s) in (\"\")"=w660) -> ("States Out"=w659:string)  [unwired: 14 in]
      }
      frame "Data: Cleanup" {
        # "Cleanup any data and references, here.\n(this is called automatically, by the Macro: Exit)"
        n261 = Unbundle By Name(w662) -> ("Core.Current VI Reference"=w665:refnum<vi>)
        n262 = Close Reference(reference=w665, error in (no error)=w664) -> (error out=w663:errorcluster)
        n263 = call <vilib>:"Add State(s) to Queue__JKI_lib_State_Machine.vi"("State(s) in (\"\")"=w667) -> ("States Out"=w666:string)  [unwired: 14 in]
      }
      frame "Data: OpenTDMS" {
        # "Open tdms file and save ref num\n(It is a separator no-op. You can make a copy of this frame to create a new Data frame)"
        n264 = call "RunIDFGV.vi"("action (write)"=enum16{"write", "read"}."read") -> ("RunID out"=w675:u16)  [unwired: 9 in, 1 out]
        n265 = Unbundle By Name(w682) -> ("SaveFilePath"=w671:path)
        n266 = Number To Decimal String(number=w675, width (-)=i16 3) -> (decimal integer string=w673:string)
        n267 = Get Date/Time In Seconds() -> (seconds since 1Jan1904=w679:timestamp)
        n268 = Format Date/Time String(time format string (%c)="%Y%m%d %H_%M", seconds (now)=w679) -> (date/time string=w672:string)  [unwired: 1 in]
        n269 = Concatenate Strings("Run" ("string"), w673, w672, ".tdms" ("string")) -> (w670:string)
        n270 = Build Path(base path=w671, name or relative path=w670) -> (appended path=w668:path)
        n271 = TDMS Open(8:w683, 10:T12."create" ("operation (0:open)"), 11:w668) -> (0:w684:errorcluster, 3:w680:refnum<k34>)  [unwired: 4 in]
        n272 = Bundle By Name(cluster=w682, "tdms file"=w680) -> (w681:T15)
        n273 = call <vilib>:"Add State(s) to Queue__JKI_lib_State_Machine.vi"("State(s) in (\"\")"=w688) -> ("States Out"=w687:string)  [unwired: 14 in]
      }
      frame "Data: SaveExpDetail" {
        # "Save 3D profile to tdms file\n(save y pixel size, raw 3D profile and processed 3D profile to file)"
        n274 = Unbundle By Name(w698) -> ("tdms file"=w697:refnum<k34>)
        n275 = TDMS Set Properties(5:"FLIm 3D Scan", 7:"System", 8:w696, 11:w697) -> (0:w692:errorcluster, 3:w693:refnum<k34>)  [unwired: 2 in, 2 out]
        n276 = Get Date/Time In Seconds() -> (seconds since 1Jan1904=w690:timestamp)
        n277 = TDMS Set Properties(5:w690, 7:"datetime", 8:w692, 11:w693) -> (0:w691:errorcluster)  [unwired: 2 in, 3 out]
        n278 = call <vilib>:"Add State(s) to Queue__JKI_lib_State_Machine.vi"("State(s) in (\"\")"=w701) -> ("States Out"=w700:string)  [unwired: 14 in]
      }
      frame "Data: SaveRaw3DProfile" {
        # "Save 3D profile to tdms file\n(save y pixel size, raw 3D profile and processed 3D profile to file)"
        n279 = Unbundle By Name(w726) -> ("tdms file"=w708:refnum<k34>, "Raw3DProfileNoY"=w723:cluster{"x(mm)":dbl, "y(mm)":dbl, "z(mm)":dbl}[], "YPixelSize(mm)"=w716:dbl)
        n280 = for {
          tunnel: w723 -> [w732] mode=indexing
          tunnel: [w731] -> w722 mode=indexing
          tunnel: [w730] -> w721 mode=indexing
          n281 = Unbundle By Name(w732) -> ("x(mm)"=w731:dbl, "z(mm)"=w730:dbl)
        }
        n282 = Build Array(w722, w721) -> (w720:dbl[][])
        n283 = TDMS Write(0:w708, 5:"Raw3DProfile" ("group name in (Untitled)"), 7:string[] ["x", "z"] ("channel name(s) in (Untitled)"), 9:w720, 11:w709) -> (4:w719:refnum<k34>, 6:w718:string, 15:w715:errorcluster)  [unwired: 1 in, 1 out]
        n284 = TDMS Set Properties(5:w716, 7:"Y pixel size", 8:w715, 10:w718, 11:w719) -> (0:w713:errorcluster, 2:w712:string, 3:w714:refnum<k34>)  [unwired: 1 in, 1 out]
        n285 = local read "Pre Scan Speed (mm/min)"() -> (w703:sgl)
        n286 = TDMS Set Properties(5:"mm", 7:"unit", 8:w713, 10:w712, 11:w714) -> (0:w706:errorcluster, 2:w705:string, 3:w707:refnum<k34>)  [unwired: 1 in, 1 out]
        n287 = TDMS Set Properties(5:w703, 7:"ScanSpeed(mm/min)", 8:w706, 10:w705, 11:w707) -> (0:w702:errorcluster)  [unwired: 1 in, 3 out]
        n288 = call <vilib>:"Add State(s) to Queue__JKI_lib_State_Machine.vi"("State(s) in (\"\")"=w729) -> ("States Out"=w728:string)  [unwired: 14 in]
      }
      frame "Data: SaveProcessed3DProfile" {
        # "Save 3D profile to tdms file\n(save y pixel size, raw 3D profile and processed 3D profile to file)"
        n289 = Unbundle By Name(w748) -> ("tdms file"=w734:refnum<k34>, "3DProfile"=w745:cluster{"x(mm)":dbl, "y(mm)":dbl, "z(mm)":dbl}[])
        n290 = for {
          tunnel: w745 -> [w755] mode=indexing
          tunnel: [w754] -> w744 mode=indexing
          tunnel: [w753] -> w743 mode=indexing
          tunnel: [w752] -> w733 mode=indexing
          n291 = Unbundle By Name(w755) -> ("x(mm)"=w754:dbl, "y(mm)"=w753:dbl, "z(mm)"=w752:dbl)
        }
        n292 = Build Array(w744, w743, w733) -> (w742:dbl[][])
        n293 = TDMS Write(0:w734, 5:"Processed3DProfile" ("group name in (Untitled)"), 7:string[] ["x", "y", "z"] ("channel name(s) in (Untitled)"), 9:w742, 11:w735) -> (4:w741:refnum<k34>, 6:w740:string, 15:w739:errorcluster)  [unwired: 1 in, 1 out]
        n294 = TDMS Set Properties(5:"mm", 7:"unit", 8:w739, 10:w740, 11:w741) -> (0:w736:errorcluster)  [unwired: 1 in, 3 out]
        n295 = call <vilib>:"Add State(s) to Queue__JKI_lib_State_Machine.vi"("State(s) in (\"\")"=w751) -> ("States Out"=w750:string)  [unwired: 14 in]
      }
      frame "Data: SaveFollowScan" {
        # "Save 3D profile to tdms file\n(save y pixel size, raw 3D profile and processed 3D profile to file)"
        n296 = Unbundle By Name(w789) -> ("tdms file"=w776:refnum<k34>, "FollowScan"=w786:cluster{"x(mm)":dbl, "y(mm)":dbl, "z(mm)":dbl}[], "FiberOffset"=w770:cluster{"x":dbl, "y":dbl}, "FollowScanZOffset(mm)"=w762:dbl, "ProbeRadius(mm)"=w757:dbl)
        n297 = for {
          tunnel: w786 -> [w796] mode=indexing
          tunnel: [w795] -> w785 mode=indexing
          tunnel: [w794] -> w784 mode=indexing
          tunnel: [w793] -> w775 mode=indexing
          n298 = Unbundle By Name(w796) -> ("x(mm)"=w795:dbl, "y(mm)"=w794:dbl, "z(mm)"=w793:dbl)
        }
        n299 = Build Array(w785, w784, w775) -> (w783:dbl[][])
        n300 = TDMS Write(0:w776, 5:"FollowScan3D" ("group name in (Untitled)"), 7:string[] ["x", "y", "z"] ("channel name(s) in (Untitled)"), 9:w783, 11:w777) -> (4:w782:refnum<k34>, 6:w781:string, 15:w780:errorcluster)  [unwired: 1 in, 1 out]
        n301 = Unbundle By Name(w770) -> ("x"=w769:dbl, "y"=w768:dbl)
        n302 = TDMS Set Properties(5:"mm", 7:"unit", 8:w780, 10:w781, 11:w782) -> (0:w772:errorcluster, 2:w773:string, 3:w774:refnum<k34>)  [unwired: 1 in, 1 out]
        n303 = Build Array(w769, w768) -> (w767:dbl[])
        n304 = TDMS Set Properties(5:w767, 7:string[] ["FiberOffSetX", "FiberOffSetY"] ("property names"), 8:w772, 10:w773, 11:w774) -> (0:w765:errorcluster, 2:w764:string, 3:w766:refnum<k34>)  [unwired: 1 in, 1 out]
        n305 = TDMS Set Properties(5:w762, 7:"FollowOffsetZ", 8:w765, 10:w764, 11:w766) -> (0:w760:errorcluster, 2:w759:string, 3:w761:refnum<k34>)  [unwired: 1 in, 1 out]
        n306 = TDMS Set Properties(5:w757, 7:"ProbeRadius", 8:w760, 10:w759, 11:w761) -> (0:w756:errorcluster)  [unwired: 1 in, 3 out]
        n307 = call <vilib>:"Add State(s) to Queue__JKI_lib_State_Machine.vi"("State(s) in (\"\")"=w792) -> ("States Out"=w791:string)  [unwired: 14 in]
      }
      frame "Data: SaveInterpedFollowScan" {
        # "Save 3D profile to tdms file\n(save y pixel size, raw 3D profile and processed 3D profile to file)"
        n308 = Unbundle By Name(w817) -> ("tdms file"=w804:refnum<k34>, "FollowScanWInter"=w814:cluster{"x(mm)":dbl, "y(mm)":dbl, "z(mm)":dbl}[], "FollowGridSize(mm)"=w798:dbl)
        n309 = for {
          tunnel: w814 -> [w824] mode=indexing
          tunnel: [w823] -> w813 mode=indexing
          tunnel: [w822] -> w812 mode=indexing
          tunnel: [w821] -> w803 mode=indexing
          n310 = Unbundle By Name(w824) -> ("x(mm)"=w823:dbl, "y(mm)"=w822:dbl, "z(mm)"=w821:dbl)
        }
        n311 = Build Array(w813, w812, w803) -> (w811:dbl[][])
        n312 = TDMS Write(0:w804, 5:"InterpedFollowScan3D" ("group name in (Untitled)"), 7:string[] ["x", "y", "z"] ("channel name(s) in (Untitled)"), 9:w811, 11:w805) -> (4:w810:refnum<k34>, 6:w809:string, 15:w808:errorcluster)  [unwired: 1 in, 1 out]
        n313 = TDMS Set Properties(5:"mm", 7:"unit", 8:w808, 10:w809, 11:w810) -> (0:w800:errorcluster, 2:w801:string, 3:w802:refnum<k34>)  [unwired: 1 in, 1 out]
        n314 = TDMS Set Properties(5:w798, 7:"GridSize(mm)", 8:w800, 10:w801, 11:w802) -> (0:w797:errorcluster)  [unwired: 1 in, 3 out]
        n315 = call <vilib>:"Add State(s) to Queue__JKI_lib_State_Machine.vi"("State(s) in (\"\")"=w820) -> ("States Out"=w819:string)  [unwired: 14 in]
      }
      frame "Data: SaveRawFollowScanData" {
        # "Save 3D profile to tdms file\n(save y pixel size, raw 3D profile and processed 3D profile to file)"
        n316 = Unbundle By Name(w849) -> ("tdms file"=w841:refnum<k34>, "RawFollowScanData"=w846:cluster{"Time(ms)":dbl, "x":dbl}[], "YPixelSize(mm)"=w837:dbl)
        n317 = for {
          tunnel: w846 -> [w855] mode=indexing
          tunnel: [w854] -> w845 mode=indexing
          tunnel: [w853] -> w844 mode=indexing
          n318 = Unbundle By Name(w855) -> ("x"=w854:dbl, "Time(ms)"=w853:dbl)
        }
        n319 = Build Array(w845, w844) -> (w843:dbl[][])
        n320 = TDMS Write(0:w841, 5:"RawFollowScanData" ("group name in (Untitled)"), 7:string[] ["x", "Time(ms)", ""] ("channel name(s) in (Untitled)"), 9:w843, 11:w842) -> (4:w840:refnum<k34>, 6:w839:string, 15:w838:errorcluster)  [unwired: 1 in, 1 out]
        n321 = local read "Follow Speed (mm/min)"() -> (w831:sgl)
        n322 = TDMS Set Properties(5:w837, 7:"Y pixel size", 8:w838, 10:w839, 11:w840) -> (0:w834:errorcluster, 2:w833:string, 3:w835:refnum<k34>)  [unwired: 1 in, 1 out]
        n323 = local read "LocationPollingStart"() -> (w825:u32)
        n324 = TDMS Set Properties(5:w831, 7:"ScanSpeed(mm/min)", 8:w834, 10:w833, 11:w835) -> (0:w829:errorcluster, 2:w826:string, 3:w830:refnum<k34>)  [unwired: 1 in, 1 out]
        n325 = TDMS Set Properties(5:w825, 7:"FollowScanStartTime", 8:w829, 10:w826, 11:w830) -> (0:w828:errorcluster)  [unwired: 1 in, 3 out]
        n326 = call <vilib>:"Add State(s) to Queue__JKI_lib_State_Machine.vi"("State(s) in (\"\")"=w852) -> ("States Out"=w851:string)  [unwired: 14 in]
      }
      frame "Data: SaveProcessedPPIXImg" {
        # "Save 3D profile to tdms file\n(save y pixel size, raw 3D profile and processed 3D profile to file)"
        n327 = Unbundle By Name(w866) -> ("tdms file"=w861:refnum<k34>, "PPIXProcessedImg"=w859:cluster{"x":dbl[], "y":dbl[], "Time(ms)":dbl[]})
        n328 = Unbundle By Name(w859) -> ("x"=w856:dbl[], "y"=w858:dbl[], "Time(ms)"=w857:dbl[])
        n329 = Build Array(w856, w858, w857) -> (w863:dbl[][])
        n330 = TDMS Write(0:w861, 5:"ProcessedFollowScanData" ("group name in (Untitled)"), 7:string[] ["x", "y", "Time(ms)"] ("channel name(s) in (Untitled)"), 9:w863, 11:w862) -> (15:w860:errorcluster)  [unwired: 1 in, 3 out]
        n331 = call <vilib>:"Add State(s) to Queue__JKI_lib_State_Machine.vi"("State(s) in (\"\")"=w869) -> ("States Out"=w868:string)  [unwired: 14 in]
      }
      frame "Data: CloseTDMS" {
        # "Close tfms file.\n(It is a separator no-op. You can make a copy of this frame to create a new Data frame)"
        n332 = Unbundle By Name(w873) -> ("tdms file"=w872:refnum<k34>)
        n333 = TDMS Close(8:w870, 11:w872) -> (0:w871:errorcluster)  [unwired: 1 out]
        n334 = call <vilib>:"Add State(s) to Queue__JKI_lib_State_Machine.vi"("State(s) in (\"\")"=w876) -> ("States Out"=w875:string)  [unwired: 14 in]
      }
      frame "Data: CreatDataFolder" {
        # "Do not put any code in this frame.\n(It is a separator no-op. You can make a copy of this frame to create a new Data frame)"
        n335 = call "DataRootPathFGV.vi"("Error In"=w877, "action (write)"=enum16{"write", "read"}."read") -> ("Error Out"=w885:errorcluster, "PathOut"=w888:path)  [unwired: 8 in]
        n336 = Build Path(base path=w888, name or relative path="3DScanData") -> (appended path=w886:path)
        n337 = call <vilib>:"Check if File or Folder Exists.vi"("error in (no error)"=w885, "path"=w886) -> ("error out"=w879:errorcluster, "file or folder exists?"=w884:bool, "dup path"=w881:path)  [unwired: 7 in]
        n338 = case shown="False" w884 {
          tunnel: w881 -> [w896 w898]
          tunnel: [w894 w898] -> w880
          tunnel: w879 -> [w895 w897]
          tunnel: [w893 w897] -> w878
          frame False {
            # "if folder not exist, creat folder"
            n339 = Create Folder(path (use dialog)=w896, error in=w895) -> (created path=w894:path, error out=w893:errorcluster)  [unwired: 1 in, 1 out]
          }
          frame True {
            # "If folder exist, do nothing"
          }
        }
        n340 = Bundle By Name(cluster=w883, "SaveFilePath"=w880) -> (w882:T15)
        n341 = call <vilib>:"Add State(s) to Queue__JKI_lib_State_Machine.vi"("State(s) in (\"\")"=w892) -> ("States Out"=w891:string)  [unwired: 14 in]
      }
      frame "---------- UI ----------" {
        # "Do not put any code in this frame.\n(It is a separator no-op. You can make a copy of this frame to create a new UI frame)"
        n342 = call <vilib>:"Add State(s) to Queue__JKI_lib_State_Machine.vi"("State(s) in (\"\")"=w903) -> ("States Out"=w902:string)  [unwired: 14 in]
      }
      frame "UI: FollowScanDone" {
        # "Do not put any code in this frame.\n(It is a separator no-op. You can make a copy of this frame to create a new UI frame)"
        n343 = property on="ShowFLImIntensity" class="Bool"("DisabledEnum"=T6."Enabled" ("Disabled")) -> ()  [unwired: 2 in, 2 out]
        n344 = call <vilib>:"Add State(s) to Queue__JKI_lib_State_Machine.vi"("State(s) in (\"\")"=w909) -> ("States Out"=w908:string)  [unwired: 14 in]
      }
      frame "UI: 3DScanDone" {
        w910 = T6."Disabled and Grayed Out" ("Disabled")
        # "Do not put any code in this frame.\n(It is a separator no-op. You can make a copy of this frame to create a new UI frame)"
        n345 = property on="Interpolate Scan" class="Bool"("DisabledEnum"=w910) -> ()  [unwired: 2 in, 2 out]
        n346 = property on="Follow Scan" class="Bool"("DisabledEnum"=w910) -> ()  [unwired: 2 in, 2 out]
        n347 = property on="ShowFLImIntensity" class="Bool"("DisabledEnum"=w910) -> ()  [unwired: 2 in, 2 out]
        n348 = property on="Plot 3D" class="Bool"("DisabledEnum"=T6."Enabled" ("Disabled")) -> ()  [unwired: 2 in, 2 out]
        n349 = property on="Calc follow scan" class="Bool"("DisabledEnum"=w910) -> ()  [unwired: 2 in, 2 out]
        n350 = property on="Remove Z outlier" class="Bool"("DisabledEnum"=w910) -> ()  [unwired: 2 in, 2 out]
        n351 = call <vilib>:"Add State(s) to Queue__JKI_lib_State_Machine.vi"("State(s) in (\"\")"=w916) -> ("States Out"=w915:string)  [unwired: 14 in]
      }
      frame "UI: StartUp" {
        w917 = T6."Disabled and Grayed Out" ("Disabled")
        # "Do not put any code in this frame.\n(It is a separator no-op. You can make a copy of this frame to create a new UI frame)"
        n352 = property on="Stage COM port" class="VISAName"("DisabledEnum"=w917) -> ()  [unwired: 2 in, 2 out]
        n353 = property on="Range Finder COM" class="VISAName"("DisabledEnum"=w917) -> ()  [unwired: 2 in, 2 out]
        n354 = property on="3DProfileScan" class="Bool"("DisabledEnum"=w917) -> ()  [unwired: 2 in, 2 out]
        n355 = property on="Plot 3D" class="Bool"("DisabledEnum"=w917) -> ()  [unwired: 2 in, 2 out]
        n356 = property on="Remove Z outlier" class="Bool"("DisabledEnum"=w917) -> ()  [unwired: 2 in, 2 out]
        n357 = property on="Interpolate Scan" class="Bool"("DisabledEnum"=w917) -> ()  [unwired: 2 in, 2 out]
        n358 = local write "Tab Control"(T2."Stage Setting" ("Tab Control")) -> ()
        n359 = property on="Calc follow scan" class="Bool"("DisabledEnum"=w917) -> ()  [unwired: 2 in, 2 out]
        n360 = property on="Follow Scan" class="Bool"("DisabledEnum"=w917) -> ()  [unwired: 2 in, 2 out]
        n361 = property on="ShowFLImIntensity" class="Bool"("DisabledEnum"=w917) -> ()  [unwired: 2 in, 2 out]
        n362 = property on="X-Axis configuration" class="Clust (strict)"("DisabledEnum"=w917) -> ()  [unwired: 2 in, 2 out]
        n363 = property on="Y-Axis configuration" class="Clust (strict)"("DisabledEnum"=w917) -> ()  [unwired: 2 in, 2 out]
        n364 = property on="Z-Axis configuration" class="Clust (strict)"("DisabledEnum"=w917) -> ()  [unwired: 2 in, 2 out]
        n365 = property on="Set Origin" class="Bool"("DisabledEnum"=w917) -> ()  [unwired: 2 in, 2 out]
        n366 = property on="Poll grbl position?" class="Bool (strict)"("DisabledEnum"=w917) -> ()  [unwired: 2 in, 2 out]
        n367 = property on="X++" class="Bool"("DisabledEnum"=w917) -> ()  [unwired: 2 in, 2 out]
        n368 = property on="X--" class="Bool"("DisabledEnum"=w917) -> ()  [unwired: 2 in, 2 out]
        n369 = property on="Y++" class="Bool"("DisabledEnum"=w917) -> ()  [unwired: 2 in, 2 out]
        n370 = property on="Y--" class="Bool"("DisabledEnum"=w917) -> ()  [unwired: 2 in, 2 out]
        n371 = property on="Z++" class="Bool"("DisabledEnum"=w917) -> ()  [unwired: 2 in, 2 out]
        n372 = property on="Z--" class="Bool"("DisabledEnum"=w917) -> ()  [unwired: 2 in, 2 out]
        n373 = property on="Hault" class="Bool"("DisabledEnum"=w917) -> ()  [unwired: 2 in, 2 out]
        n374 = property on="GoToZero" class="Bool"("DisabledEnum"=w917) -> ()  [unwired: 2 in, 2 out]
        n375 = property on="Home" class="Bool"("DisabledEnum"=w917) -> ()  [unwired: 2 in, 2 out]
        n376 = call <vilib>:"Add State(s) to Queue__JKI_lib_State_Machine.vi"("State(s) in (\"\")"=w923) -> ("States Out"=w922:string)  [unwired: 14 in]
      }
      frame "UI: Exit" {
        w924 = T6."Enabled" ("Disabled")
        # "Do not put any code in this frame.\n(It is a separator no-op. You can make a copy of this frame to create a new UI frame)"
        n377 = property on="Stage COM port" class="VISAName"("DisabledEnum"=w924) -> ()  [unwired: 2 in, 2 out]
        n378 = property on="Range Finder COM" class="VISAName"("DisabledEnum"=w924) -> ()  [unwired: 2 in, 2 out]
        n379 = property on="X-Axis configuration" class="Clust (strict)"("DisabledEnum"=w924) -> ()  [unwired: 2 in, 2 out]
        n380 = property on="Y-Axis configuration" class="Clust (strict)"("DisabledEnum"=w924) -> ()  [unwired: 2 in, 2 out]
        n381 = property on="Z-Axis configuration" class="Clust (strict)"("DisabledEnum"=w924) -> ()  [unwired: 2 in, 2 out]
        n382 = call <vilib>:"Add State(s) to Queue__JKI_lib_State_Machine.vi"("State(s) in (\"\")"=w929) -> ("States Out"=w928:string)  [unwired: 14 in]
      }
      frame "UI: SysReady" {
        # "System finished start up and ready for use\n(It is a separator no-op. You can make a copy of this frame to create a new UI frame)"
        n383 = call <vilib>:"Add State(s) to Queue__JKI_lib_State_Machine.vi"("State(s) in (\"\")"=w934) -> ("States Out"=w933:string)  [unwired: 14 in]
      }
      frame "UI: Update" {
        # "Do not put any code in this frame.\n(It is a separator no-op. You can make a copy of this frame to create a new UI frame)"
        n384 = Unbundle By Name(w939) -> ("Sys Status"=w937:T1, "StageHomed?"=w935:bool)
        "Sys Status" <- w937
        n385 = Unbundle By Name(w937) -> ("Stage"=w936:bool)
        n386 = case shown="True" w935 {
          frame False {
          }
          frame True {
            w943 = T6."Enabled" ("Disabled")
            n387 = property on="GoToZero" class="Bool"("DisabledEnum"=w943) -> ()  [unwired: 2 in, 2 out]
            n388 = property on="3DProfileScan" class="Bool"("DisabledEnum"=w943) -> ()  [unwired: 2 in, 2 out]
          }
        }
        n389 = case shown="True" w936 {
          frame False {
          }
          frame True {
            w944 = T6."Enabled" ("Disabled")
            n390 = property on="Set Origin" class="Bool"("DisabledEnum"=w944) -> ()  [unwired: 2 in, 2 out]
            n391 = property on="Poll grbl position?" class="Bool (strict)"("DisabledEnum"=w944) -> ()  [unwired: 2 in, 2 out]
            n392 = property on="X++" class="Bool"("DisabledEnum"=w944) -> ()  [unwired: 2 in, 2 out]
            n393 = property on="X--" class="Bool"("DisabledEnum"=w944) -> ()  [unwired: 2 in, 2 out]
            n394 = property on="Y++" class="Bool"("DisabledEnum"=w944) -> ()  [unwired: 2 in, 2 out]
            n395 = property on="Y--" class="Bool"("DisabledEnum"=w944) -> ()  [unwired: 2 in, 2 out]
            n396 = property on="Z++" class="Bool"("DisabledEnum"=w944) -> ()  [unwired: 2 in, 2 out]
            n397 = property on="Z--" class="Bool"("DisabledEnum"=w944) -> ()  [unwired: 2 in, 2 out]
            n398 = property on="Hault" class="Bool"("DisabledEnum"=w944) -> ()  [unwired: 2 in, 2 out]
            n399 = property on="Home" class="Bool"("DisabledEnum"=w944) -> ()  [unwired: 2 in, 2 out]
          }
        }
        n400 = call <vilib>:"Add State(s) to Queue__JKI_lib_State_Machine.vi"("State(s) in (\"\")"=w942) -> ("States Out"=w941:string)  [unwired: 14 in]
      }
      frame "UI: Initialize" {
        # "Initialize the User Interface, here.\n(this is called automatically, by the Macro: Init)"
        n401 = call <vilib>:"Add State(s) to Queue__JKI_lib_State_Machine.vi"("State(s) in (\"\")"=w949) -> ("States Out"=w948:string)  [unwired: 14 in]
      }
      frame "UI: Cursor Set" {
        # "Argument"
        # "Set and Unset Cursor Busy.\n(Usage: \"UI: Cursor Set >> Busy|Idle\")"
        n402 = case shown="\"Idle\", Default" w951 {
          tunnel: w953 -> [w958 w960]
          tunnel: [w957 w959] -> w952
          frame "Idle", Default {
            n403 = call <vilib>:"Unset Busy.vi"("error in (no error)"=w958) -> ("error out"=w957:errorcluster)  [unwired: 10 in]
          }
          frame "Busy" {
            n404 = call <vilib>:"Set Busy.vi"("error in (no error)"=w960) -> ("error out"=w959:errorcluster)  [unwired: 9 in, 1 out]
          }
        }
        n405 = call <vilib>:"Add State(s) to Queue__JKI_lib_State_Machine.vi"("State(s) in (\"\")"=w956) -> ("States Out"=w955:string)  [unwired: 14 in]
      }
      frame "UI: Front Panel State" {
        # "Argument"
        # "Set Front Panel Open or Closed\n(Usage: \"UI: Front Panel State >> Open|Close\")"
        n406 = Unbundle By Name(w964) -> ("Core.Current VI Reference"=w963:refnum<vi>)
        n407 = case shown="\"Open\", \"Standard\", Default" w962 {
          tunnel: w966 -> [w974 w989 w1000 w1013 w1026]
          tunnel: [w976 w990 w1002 w1015 w1028] -> w965
          tunnel: w963 -> [w975 w987 w1001 w1014 w1027]
          frame "Open", "Standard", Default {
            w969 = T10."Standard" ("State")
            n408 = property class="VI"(reference=w975, error in=w974) -> (reference out=w972:refnum<vi>, error out=w973:errorcluster, "FP.State"=w971:T10)
            n409 = Not Equal?(x=w971, y=w969) -> (x != y?=w970:bool)
            n410 = case shown="True" w970 {
              tunnel: [w980 w982] -> w976
              tunnel: w973 -> [w979 w982]
              tunnel: w972 -> [w978 _]
              tunnel: w969 -> [w977 _]
              frame True {
                n411 = invoke class="VI" method="FP.Open"(reference=w978, error in=w979, "Activate"=TRUE, "State"=w977) -> (error out=w980:errorcluster)  [unwired: 1 in, 4 out]
              }
              frame False {
              }
            }
          }
          frame "Close", "Closed" {
            n412 = property class="VI"(reference=w987, error in=w989) -> (reference out=w986:refnum<vi>, error out=w988:errorcluster, "FP.State"=w984:T10)
            n413 = Not Equal?(x=w984, y=T10."Closed" ("Front Panel Window:State")) -> (x != y?=w983:bool)
            n414 = case shown="True" w983 {
              tunnel: [w991 w994] -> w990
              tunnel: w988 -> [w991 w993]
              tunnel: w986 -> [_ w992]
              frame False {
              }
              frame True {
                n415 = invoke class="VI" method="FP.Close"(reference=w992, error in=w993) -> (error out=w994:errorcluster)  [unwired: 1 in, 2 out]
              }
            }
          }
          frame "Hidden", "Hide" {
            w995 = T10."Hidden" ("State")
            n416 = property class="VI"(reference=w1001, error in=w1000) -> (reference out=w998:refnum<vi>, error out=w999:errorcluster, "FP.State"=w997:T10)
            n417 = Not Equal?(x=w997, y=w995) -> (x != y?=w996:bool)
            n418 = case shown="True" w996 {
              tunnel: [w1006 w1007] -> w1002
              tunnel: w999 -> [w1005 w1007]
              tunnel: w998 -> [w1004 _]
              tunnel: w995 -> [w1003 _]
              frame True {
                n419 = invoke class="VI" method="FP.Open"(reference=w1004, error in=w1005, "State"=w1003) -> (error out=w1006:errorcluster)  [unwired: 2 in, 4 out]
              }
              frame False {
              }
            }
          }
          frame "Minimize", "Minimized" {
            w1008 = T10."Minimized" ("State")
            n420 = property class="VI"(reference=w1014, error in=w1013) -> (reference out=w1011:refnum<vi>, error out=w1012:errorcluster, "FP.State"=w1010:T10)
            n421 = Not Equal?(x=w1010, y=w1008) -> (x != y?=w1009:bool)
            n422 = case shown="True" w1009 {
              tunnel: [w1019 w1020] -> w1015
              tunnel: w1012 -> [w1018 w1020]
              tunnel: w1011 -> [w1017 _]
              tunnel: w1008 -> [w1016 _]
              frame True {
                n423 = invoke class="VI" method="FP.Open"(reference=w1017, error in=w1018, "State"=w1016) -> (error out=w1019:errorcluster)  [unwired: 2 in, 4 out]
              }
              frame False {
              }
            }
          }
          frame "Maximize", "Maximized" {
            w1021 = T10."Maximized" ("State")
            n424 = property class="VI"(reference=w1027, error in=w1026) -> (reference out=w1024:refnum<vi>, error out=w1025:errorcluster, "FP.State"=w1023:T10)
            n425 = Not Equal?(x=w1023, y=w1021) -> (x != y?=w1022:bool)
            n426 = case shown="True" w1022 {
              tunnel: [w1032 w1033] -> w1028
              tunnel: w1025 -> [w1031 w1033]
              tunnel: w1024 -> [w1030 _]
              tunnel: w1021 -> [w1029 _]
              frame True {
                n427 = invoke class="VI" method="FP.Open"(reference=w1030, error in=w1031, "State"=w1029) -> (error out=w1032:errorcluster)  [unwired: 2 in, 4 out]
              }
              frame False {
              }
            }
          }
        }
        n428 = call <vilib>:"Add State(s) to Queue__JKI_lib_State_Machine.vi"("State(s) in (\"\")"=w968) -> ("States Out"=w967:string)  [unwired: 14 in]
      }
      frame "---------- Stage ----------" {
        # "Template Separator\n(You can make a copy of, or modify, this frame)"
        n429 = call <vilib>:"Add State(s) to Queue__JKI_lib_State_Machine.vi"("State(s) in (\"\")"=w1038) -> ("States Out"=w1037:string)  [unwired: 14 in]
      }
      frame "Stage: Initialize" {
        # "Initialize stage controler\n(Open connection and check)"
        n430 = call "Initialize Serial Port.vi"("VISA resource name"="Stage COM port", "baud rate (115200)"=u32 115200, "error in (no error)"=w1048) -> ("error out"=w1045:errorcluster)  [unwired: 12 in]
        n431 = call "Get Version.vi"("error in (no error)"=w1045) -> ("Version information"=→"Version information":string, "error out"=w1039:errorcluster)  [unwired: 12 in, 1 out]
        n432 = case shown="No Error" w1039 {
          selector: w1039 -> [w1051 _]
          tunnel: [w1051 w1052] -> w1044
          frame No Error {
          }
          frame Error {
            # "If grbl respond is wrong"
            n433 = xnode "Error Ring"() -> ("error out"=w1052:errorcluster)
          }
        }
        n434 = case shown="No Error" w1039 {
          tunnel: [w1060 w1062] -> w1047
          tunnel: w1040 -> [w1059 w1062]
          tunnel: "Stage COM port" -> [w1058 _]
          frame No Error {
            n435 = Bundle By Name(cluster=w1059, "Sys Status.Stage"=TRUE, "StageCOM"=w1058) -> (w1060:T15)
          }
          frame Error {
          }
        }
        n436 = call <vilib>:"Add State(s) to Queue__JKI_lib_State_Machine.vi"("State(s) in (\"\")"=w1050) -> ("States Out"=w1049:string)  [unwired: 14 in]
      }
      frame "Stage: Reset" {
        # "Reset grbl\n(Ctrl+x)"
        n437 = call "Reset.vi"("error in (no error)"=w1064) -> ("error out"=w1065:errorcluster)  [unwired: 14 in]
        n438 = call <vilib>:"Add State(s) to Queue__JKI_lib_State_Machine.vi"("State(s) in (\"\")"=w1068) -> ("States Out"=w1067:string)  [unwired: 14 in]
      }
      frame "Stage: Config" {
        # "set G code parser and default speed 2000"
        # "Initialize stage controler and set default configuration\n()"
        n439 = call "Config IO.vi"("Pulse time us"=u32 3, "Soft limit enable"=TRUE, "Hard limit enable"=TRUE, "Step idle delay ms (255 keep)"=u8 25, "Step pulse invert"=T14 {"Reverse X"=FALSE, "Reverse Y"=FALSE, "Reverse Z"=FALSE}, "Axis direction"=T14 {"Reverse X"=TRUE, "Reverse Y"=TRUE, "Reverse Z"=TRUE}, "error in (no error)"=w1079, "Pins direction"=T13 {"Invert enable pin"=FALSE, "Invert limit pin"=FALSE, "Invert probe pin"=FALSE}) -> ("error out"=w1097:errorcluster)  [unwired: 7 in]
        n440 = call "Config Axis.vi"("X-Axis configuration"="X-Axis configuration", "Y-Axis configuration"="Y-Axis configuration", "Z-Axis configuration"="Z-Axis configuration", "error in (no error)"=w1097) -> ("error out"=w1096:errorcluster)  [unwired: 11 in]
        n441 = call "Config Home.vi"("Homing direction invert"=T14 {"Reverse X"=TRUE, "Reverse Y"=TRUE, "Reverse Z"=TRUE}, "Homing cycle enable"=TRUE, "Homing locate feed rate\tmm/min"=u32 100 ("Homing locate feed rate\tmm/min"), "Homing search seek rate\tmm/min"=u32 3000 ("Homing search seek rate\tmm/min"), "Homing switch debounce delay\tms"=u32 25 ("Homing switch debounce delay\tms"), "error in (no error)"=w1096, "Homing switch pull-off distance\tmm"=u32 2 ("Homing switch pull-off distance\tmm")) -> ("error out"=w1095:errorcluster)  [unwired: 8 in]
        n442 = call "Release Lock from Alarm.vi"("error in (no error)"=w1095) -> ("error out"=w1094:errorcluster)  [unwired: 14 in]
        n443 = call "Get Configuration.vi"("error in (no error)"=w1094) -> ("Config"=→"Current Config":string, "error out"=w1075:errorcluster)  [unwired: 13 in]
        n444 = Concatenate Strings("G1F2000" ("Data to write"), "\r") -> (w1071:string)
        n445 = call "Send-Receive Serial Port.vi"("Data to write"=w1071, "error in (no error)"=w1075) -> ("error out"=w1074:errorcluster)  [unwired: 12 in, 1 out]
        n446 = call <vilib>:"Add State(s) to Queue__JKI_lib_State_Machine.vi"("State(s) in (\"\")"=w1099) -> ("States Out"=w1098:string)  [unwired: 14 in]
      }
      frame "Stage: Home" {
        # "Home Stage\n(You can make a copy of, or modify, this frame)"
        n447 = Two Button Dialog(message="Stage will home, please retrack fiber probe and make sure no object is in its way!", 1:"Cancel" ("F button name (\"Cancel\")"), 2:"Confirm" ("T button name (\"OK\")")) -> (T button?=w1100:bool)
        n448 = case shown="True" w1100 {
          tunnel: [w1114 w1124] -> w1108
          tunnel: [w1113 w1123] -> w1107
          tunnel: w1106 -> [w1113 w1122]
          tunnel: w1104 -> [w1114 w1121]
          frame False {
            n449 = One Button Dialog(message="You must home stage before doing any scanning! Some function of the program is now disabled!", button name ("OK")="Confirm") -> ()  [unwired: 1 out]
          }
          frame True {
            # "Update origin"
            n450 = call <vilib>:"Set Busy.vi"("error in (no error)"=w1121) -> ("error out"=w1116:errorcluster)  [unwired: 9 in, 1 out]
            n451 = call "Go home.vi"("Maximum wait time (45sec)"=30, "error in (no error)"=w1116) -> ("error out"=w1120:errorcluster)  [unwired: 13 in]
            n452 = call <vilib>:"Unset Busy.vi"("error in (no error)"=w1120) -> ("error out"=w1115:errorcluster)  [unwired: 10 in]
            n453 = Unbundle By Name(w1120) -> ("status"=w1119:bool)
            n454 = call "Get Status.vi"("error in (no error)"=w1115) -> ("Current position"=w1117:cluster{"X":sgl, "Y":sgl, "Z":sgl}, "error out"=w1124:errorcluster)  [unwired: 10 in, 3 out]
            "Stage Home MPos" <- w1117
            n455 = Not(x=w1119) -> (.not. x?=w1118:bool)
            n456 = local write "Current Machine Pos"(w1117) -> ()
            n457 = Bundle By Name(cluster=w1122, "StageHomed?"=w1118, "HomeMposOrigin"=w1117) -> (w1123:T15)
          }
        }
        n458 = call <vilib>:"Add State(s) to Queue__JKI_lib_State_Machine.vi"("State(s) in (\"\")"=w1110) -> ("States Out"=w1109:string)  [unwired: 14 in]
      }
      frame "Stage: GoToZero" {
        # "Go to scanning origin marked on the platform\n(Go to scanning start and set original position)"
        n459 = Unbundle By Name(w1127) -> ("StageHomed?"=w1126:bool)
        n460 = case shown="True" w1126 {
          tunnel: w1131 -> [w1137 w1144]
          tunnel: [w1137 w1143] -> w1130
          tunnel: [w1136 w1142] -> w1129
          tunnel: w1127 -> [w1136 w1140]
          frame False {
            # "stage not homed, do nothing"
            n461 = One Button Dialog(message="Stage not homed! Could not go to scan origin marked on stage platform! Please home stage and go to scan origin manually using the stage control.", button name ("OK")="Confirm") -> ()  [unwired: 1 out]
          }
          frame True {
            # "If stage is homed, move to scan origin"
            n462 = One Button Dialog(message="System will now go to scan starting point marked on the stage. Please make sure the stage is clear of any object.", button name ("OK")="Confirm" ("T button name (\"OK\")")) -> (true=w1138:bool)
            n463 = case shown="True" w1138 {
              tunnel: w1144 -> [w1146 w1157]
              tunnel: [w1146 w1150] -> w1143
              tunnel: [w1145 w1149] -> w1142
              tunnel: w1140 -> [w1145 w1147]
              frame False {
                # "user not confirmed, do nothing"
              }
              frame True {
                # "reset encoder"
                # "User confirm moving to scan origin"
                n464 = call "Get Status.vi"("error in (no error)"=w1157) -> ("Status"=w1161:T9, "error out"=w1158:errorcluster)  [unwired: 10 in, 3 out]
                n465 = Equal?(x=Status."Idle" ("Status"), y=w1161) -> (x = y?=w1159:bool)
                n466 = case shown="True" w1159 {
                  tunnel: w1158 -> [w1163 w1172]
                  tunnel: [w1163 w1164] -> w1151
                  frame False {
                    n467 = One Button Dialog(message="Could not go to starting point. ") -> ()  [unwired: 1 in, 1 out]
                  }
                  frame True {
                    n468 = call <vilib>:"Set Busy.vi"("error in (no error)"=w1172) -> ("error out"=w1165:errorcluster)  [unwired: 9 in, 1 out]
                    n469 = call "Go to Position.vi"("X (mm)"=sgl 23.0, "Speed (2000 mm/min)"=sgl 3000.0 ("Speed (mm/min)"), "Overwright speed? (F)"=TRUE, "Y (mm)"=sgl 72.0, "Z (mm)"=sgl 0.0, "error in (no error)"=w1165) -> ("error out"=w1168:errorcluster)  [unwired: 9 in]
                    n470 = call <vilib>:"Unset Busy.vi"("error in (no error)"=w1168) -> ("error out"=w1164:errorcluster)  [unwired: 10 in]
                  }
                }
                n471 = call "Get Status.vi"("error in (no error)"=w1151) -> ("Current position"=w1148:cluster{"X":sgl, "Y":sgl, "Z":sgl}, "error out"=w1152:errorcluster)  [unwired: 10 in, 3 out]
                n472 = Bundle By Name(cluster=w1147, "ScanOrigin"=w1148) -> (w1149:T15)
                n473 = call "LabJack_FGV_T4.vi"("Operation(Read)"=enum16{"Write", "Read"}."Read" ("Operation"), "error in (no error)"=w1152) -> ("error out"=w1155:errorcluster, "Read data"=w1154:i32)  [unwired: 8 in]
                n474 = call "LJM_eReadName.vi"("Handle In"=w1154, "Name"="DIO4_EF_READ_A_AND_RESET", "error in"=w1155) -> ("error out"=w1150:errorcluster)  [unwired: 10 in, 2 out]
                n475 = local write "Scan Origin MPos"(w1148) -> ()
              }
            }
          }
        }
        n476 = call <vilib>:"Add State(s) to Queue__JKI_lib_State_Machine.vi"("State(s) in (\"\")"=w1133) -> ("States Out"=w1132:string)  [unwired: 14 in]
      }
      frame "Stage: SendCommand" {
        # "Template Separator\n(You can make a copy of, or modify, this frame)"
        n477 = call "Send-Receive Serial Port.vi"("Data to write"=w1174, "error in (no error)"=w1175) -> ("error out"=w1176:errorcluster)  [unwired: 12 in, 1 out]
        n478 = call <vilib>:"Add State(s) to Queue__JKI_lib_State_Machine.vi"("State(s) in (\"\")"=w1179) -> ("States Out"=w1178:string)  [unwired: 14 in]
      }
      frame "Stage: Close" {
        # "Close Stage connection\n(You can make a copy of, or modify, this frame)"
        n479 = Unbundle By Name(w1181) -> ("Sys Status.Stage"=w1183:bool)
        n480 = case shown="True" w1183 {
          tunnel: [w1189 w1194] -> w1185
          tunnel: w1184 -> [w1189 w1193]
          tunnel: w1181 -> [w1188 w1192]
          tunnel: [w1188 w1190] -> w1182
          frame False {
          }
          frame True {
            n481 = Bundle By Name(cluster=w1192, "Sys Status.Stage"=FALSE ("Sys Status.Stage COM")) -> (w1190:T15)
            n482 = call "Close Serial Port.vi"("error in (no error)"=w1193) -> ("error out"=w1194:errorcluster)  [unwired: 14 in]
          }
        }
        n483 = call <vilib>:"Add State(s) to Queue__JKI_lib_State_Machine.vi"("State(s) in (\"\")"=w1187) -> ("States Out"=w1186:string)  [unwired: 14 in]
      }
      frame "---------- AccuRange ----------" {
        # "Template Separator\n(You can make a copy of, or modify, this frame)"
        n484 = call <vilib>:"Add State(s) to Queue__JKI_lib_State_Machine.vi"("State(s) in (\"\")"=w1199) -> ("States Out"=w1198:string)  [unwired: 14 in]
      }
      frame "AccuRange: Initialize" {
        w1212 = u16 0 items=["None", "XON/XOFF", "RTS/CTS", "XON/XOFF & RTS/CTS", "DTR/DSR", "XON/XOFF & DTR/DSR"] ("flow control (0:none)")
        # "clear VISA buffer"
        # "Open AccuRange COM port\n(You can make a copy of, or modify, this frame)"
        n485 = call-poly "VISA Configure Serial Port"("VISA resource name"="Range Finder COM", "termination char\n(0xA = '\\n' = LF)"=u8 255 ("termination char\n(0xA = '\\n' = LF)"), "Enable Termination\nChar (T)"=TRUE ("Enable Termination\nChar (T)"), "baud rate (9600)"=u32 115200, "error in (no error)"=w1211, "flow control (0:none)"=w1212) -> ("VISA resource name out"=w1207:refnum<visa-resource-name>, "error out"=w1205:errorcluster)  [unwired: 8 in]
        n486 = VISA Clear(VISA resource name=w1207, error in (no error)=w1205) -> (VISA resource name out=w1206:refnum<visa-resource-name>, error out=w1204:errorcluster)
        n487 = case shown="Error" w1204 {
          selector: w1204 -> [w1216 _]
          tunnel: w1206 -> [w1219 _]
          tunnel: w1209 -> [w1218 w1222]
          tunnel: [w1217 w1222] -> w1208
          tunnel: [w1216 w1221] -> w1200
          frame No Error {
            n488 = Bundle By Name(cluster=w1218, "RangeCOM"=w1219, "Sys Status.RangerFinder"=TRUE) -> (w1217:T15)
          }
          frame Error {
            n489 = xnode "Error Ring"() -> ("error out"=w1221:errorcluster)
          }
        }
        n490 = call <vilib>:"Add State(s) to Queue__JKI_lib_State_Machine.vi"("State(s) in (\"\")"=w1215) -> ("States Out"=w1214:string)  [unwired: 14 in]
      }
      frame "AccuRange: Config" {
        # "Config range finder\n(You can make a copy of, or modify, this frame)"
        n491 = Unbundle By Name(w1245) -> ("RangeCOM"=w1231:refnum<visa-resource-name>)
        n492 = VISA Write(VISA resource name=w1231, write buffer="S80.X5.", error in (no error)=w1230) -> (VISA resource name out=w1244:refnum<visa-resource-name>, error out=w1235:errorcluster)  [unwired: 1 out]
        n493 = VISA Write(VISA resource name=w1244, write buffer="N.", error in (no error)=w1235) -> (VISA resource name out=w1236:refnum<visa-resource-name>, error out=w1234:errorcluster)  [unwired: 1 out]
        n494 = VISA Write(VISA resource name=w1236, write buffer="L1.", error in (no error)=w1234) -> (VISA resource name out=w1237:refnum<visa-resource-name>, error out=w1233:errorcluster)  [unwired: 1 out]
        n495 = VISA Write(VISA resource name=w1237, write buffer="A2.", error in (no error)=w1233) -> (VISA resource name out=w1238:refnum<visa-resource-name>, error out=w1232:errorcluster)  [unwired: 1 out]
        n496 = VISA Write(VISA resource name=w1238, write buffer="P1.", error in (no error)=w1232) -> (error out=w1229:errorcluster)  [unwired: 2 out]
        n497 = call <vilib>:"Add State(s) to Queue__JKI_lib_State_Machine.vi"("State(s) in (\"\")"=w1247) -> ("States Out"=w1246:string)  [unwired: 14 in]
      }
      frame "AccuRange: Start" {
        # "6"
        # "5"
        # "4"
        # "3"
        # "2"
        # "1"
        # "1. Start measurement\n2. Stop data streaming\n3. Flush read buffer to sync\n4. Restart streaming\n5. Set ranger finder loop stop flag\n6. Send user event to start loop"
        # "Start range finder\n(You can make a copy of, or modify, this frame)"
        n498 = Unbundle By Name(w1268) -> ("RangeCOM"=w1262:refnum<visa-resource-name>)
        n499 = Build Array(u8 19) -> (w1259:u8[])
        n500 = Byte Array To String(unsigned byte array=w1259) -> (string=w1256:string)
        n501 = Build Array(u8 17) -> (w1255:u8[])
        n502 = VISA Write(VISA resource name=w1262, write buffer="H1.", error in (no error)=w1261) -> (VISA resource name out=w1257:refnum<visa-resource-name>, error out=w1265:errorcluster)  [unwired: 1 out]
        n503 = Byte Array To String(unsigned byte array=w1255) -> (string=w1252:string)
        n504 = VISA Write(VISA resource name=w1257, write buffer=w1256, error in (no error)=w1265) -> (VISA resource name out=w1250:refnum<visa-resource-name>, error out=w1258:errorcluster)  [unwired: 1 out]
        n505 = VISA Flush I/O Buffer(VISA resource name=w1250, error in (no error)=w1258) -> (VISA resource name out=w1249:refnum<visa-resource-name>, error out=w1251:errorcluster)  [unwired: 1 in]
        n506 = VISA Write(VISA resource name=w1249, write buffer=w1252, error in (no error)=w1251) -> (error out=w1253:errorcluster)  [unwired: 2 out]
        n507 = flat-sequence {
          tunnel: w1253 -> [w1272]
          tunnel: [w1272] -> w1264
          frame #0 {
            n508 = local write "AccuRangeLoopStopFlag"(FALSE ("Stop Read")) -> ()
          }
        }
        n509 = Generate User Event(user event=w1267, event data cluster=TRUE ("event data"), error in=w1264) -> (error out=w1263:errorcluster)  [unwired: 1 in, 1 out]
        n510 = call <vilib>:"Add State(s) to Queue__JKI_lib_State_Machine.vi"("State(s) in (\"\")"=w1271) -> ("States Out"=w1270:string)  [unwired: 14 in]
      }
      frame "AccuRange: Stop" {
        # "stop read before turn off laser ranger. Otherwise cause VISA error and COM port can not be closed."
        # "Stop range finder\n(You can make a copy of, or modify, this frame)"
        n511 = Unbundle By Name(w1282) -> ("RangeCOM"=w1281:refnum<visa-resource-name>, "Sys Status.RangerFinder"=w1275:bool)
        n512 = flat-sequence {
          tunnel: w1280 -> [w1294]
          tunnel: [w1294] -> w1279
          frame #0 {
            n513 = local write "AccuRangeLoopStopFlag"(TRUE ("Stop Read")) -> ()
          }
        }
        n514 = call <userlib>:"Wait (ms)__ogtk.vi"("error in (no error)"=w1279, "milliseconds to wait"=u32 200) -> ("error out"=w1277:errorcluster)  [unwired: 8 in, 1 out]
        n515 = case shown="True" w1275 {
          tunnel: w1281 -> [_ w1292]
          tunnel: [w1285 w1289] -> w1278
          tunnel: w1277 -> [w1285 w1286]
          frame False {
          }
          frame True {
            n516 = VISA Write(VISA resource name=w1292, write buffer="H2.", error in (no error)=w1286) -> (VISA resource name out=w1291:refnum<visa-resource-name>, error out=w1290:errorcluster)  [unwired: 1 out]
            n517 = call <userlib>:"Wait Until Next ms Multiple__ogtk.vi"("error in (no error)"=w1290, "milliseconds to wait"=u32 500) -> ("error out"=w1288:errorcluster)  [unwired: 8 in, 1 out]
            n518 = VISA Clear(VISA resource name=w1291, error in (no error)=w1288) -> (error out=w1289:errorcluster)  [unwired: 1 out]
          }
        }
        n519 = call <vilib>:"Add State(s) to Queue__JKI_lib_State_Machine.vi"("State(s) in (\"\")"=w1284) -> ("States Out"=w1283:string)  [unwired: 14 in]
      }
      frame "AccuRange: Close" {
        # "Template Separator\n(You can make a copy of, or modify, this frame)"
        n520 = Unbundle By Name(w1297) -> ("RangeCOM"=w1299:refnum<visa-resource-name>, "Sys Status.RangerFinder"=w1302:bool)
        n521 = case shown="True" w1302 {
          tunnel: w1300 -> [w1306 w1308]
          tunnel: [w1306 w1314] -> w1301
          tunnel: w1299 -> [_ w1310]
          tunnel: w1297 -> [w1305 w1313]
          tunnel: [w1305 w1312] -> w1298
          frame False {
            # "If COM is not open, do nothing"
          }
          frame True {
            # "If COM is open, close it"
            n522 = VISA Clear(VISA resource name=w1310, error in (no error)=w1308) -> (VISA resource name out=w1309:refnum<visa-resource-name>, error out=w1307:errorcluster)
            n523 = VISA Close(VISA resource name=w1309, error in (no error)=w1307) -> (error out=w1314:errorcluster)
            n524 = Bundle By Name(cluster=w1313, "Sys Status.RangerFinder"=FALSE) -> (w1312:T15)
          }
        }
        n525 = call <vilib>:"Add State(s) to Queue__JKI_lib_State_Machine.vi"("State(s) in (\"\")"=w1304) -> ("States Out"=w1303:string)  [unwired: 14 in]
      }
      frame "---------- Utility ----------" {
        # "Template Separator\n(You can make a copy of, or modify, this frame)"
        n526 = call <vilib>:"Add State(s) to Queue__JKI_lib_State_Machine.vi"("State(s) in (\"\")"=w1319) -> ("States Out"=w1318:string)  [unwired: 14 in]
      }
      frame "Utility: DestroyQueue" {
        # "Template Separator\n(You can make a copy of, or modify, this frame)"
        n527 = Obtain Queue(name (unnamed)="FLImData", element data type=cluster{"PPIXInt":dbl, "x":dbl} {"PPIXInt"=0.0, "x"=0.0}, error in (no error)=w1321) -> (queue out=w1324:refnum<queue>, error out=w1323:errorcluster)  [unwired: 2 in, 1 out]
        n528 = Release Queue(queue=w1324, error in (no error)=w1323) -> (error out=w1322:errorcluster)  [unwired: 1 in, 2 out]
        n529 = call <vilib>:"Add State(s) to Queue__JKI_lib_State_Machine.vi"("State(s) in (\"\")"=w1329) -> ("States Out"=w1328:string)  [unwired: 14 in]
      }
      frame "Utility: Plot3D" {
        # "Template Separator\n(You can make a copy of, or modify, this frame)"
        n530 = Unbundle By Name(w1335) -> ("3DProfileToPlot"=w1334:cluster{"x(mm)":dbl, "y(mm)":dbl, "z(mm)":dbl}[])
        n531 = for {
          tunnel: w1334 -> [w1343] mode=indexing
          tunnel: [w1342] -> w1333 mode=indexing
          tunnel: [w1341] -> w1332 mode=indexing
          tunnel: [w1340] -> w1331 mode=indexing
          n532 = Unbundle By Name(w1343) -> ("x(mm)"=w1342:dbl, "y(mm)"=w1341:dbl, "z(mm)"=w1340:dbl)
        }
        n533 = call-poly <vilib>:"Plot Helper.vi"("z vector"=w1331, "y vector"=w1332, "x vector"=w1333) -> ("3D Plot lvclass Array out"=→"3D Profile":refnum<class "3D Plot Datatype.lvclass">[])  [unwired: 3 in, 5 out]
        n534 = call <vilib>:"Add State(s) to Queue__JKI_lib_State_Machine.vi"("State(s) in (\"\")"=w1339) -> ("States Out"=w1338:string)  [unwired: 14 in]
      }
      frame "Utility: Dewelling" {
        # "Template Separator\n(e.x. Dewelling >> 1000)"
        n535 = Decimal String To Number(string=w1346) -> (number=w1345:i32)  [unwired: 2 in, 1 out]
        n536 = Wait (ms)(milliseconds to wait=w1345) -> ()  [unwired: 1 out]
        n537 = call <vilib>:"Add State(s) to Queue__JKI_lib_State_Machine.vi"("State(s) in (\"\")"=w1350) -> ("States Out"=w1349:string)  [unwired: 14 in]
      }
      frame "---------- LJT4 ----------" {
        # "Template Separator\n(You can make a copy of, or modify, this frame)"
        n538 = call <vilib>:"Add State(s) to Queue__JKI_lib_State_Machine.vi"("State(s) in (\"\")"=w1355) -> ("States Out"=w1354:string)  [unwired: 14 in]
      }
      frame "LJT4: Initialize" {
        # "Open Connection to T4\n(You can make a copy of, or modify, this frame)"
        n539 = call "LJ_Open.vi"("error in"=w1360, "DeviceType"="LJM_dtT4") -> ("error out"=w1357:errorcluster, "Success?"=w1356:bool, "Handle Out"=w1358:i32)  [unwired: 7 in]
        n540 = call "LabJack_FGV_T4.vi"("Operation(Read)"=enum16{"Write", "Read"}."Write" ("Operation"), "error in (no error)"=w1357, "Write data"=w1358) -> ("error out"=w1364:errorcluster)  [unwired: 7 in, 1 out]
        n541 = Bundle By Name(cluster=w1362, "Sys Status.T4"=w1356) -> (w1363:T15)
        n542 = call <vilib>:"Add State(s) to Queue__JKI_lib_State_Machine.vi"("State(s) in (\"\")"=w1367) -> ("States Out"=w1366:string)  [unwired: 14 in]
      }
      frame "LJT4: RestEncoder" {
        # "Reset encoder \n(by read DIO4_EF_READ_A_AND_RESET)"
        n543 = call "LabJack_FGV_T4.vi"("Operation(Read)"=enum16{"Write", "Read"}."Read" ("Operation"), "error in (no error)"=w1368) -> ("error out"=w1373:errorcluster, "Read data"=w1372:i32)  [unwired: 8 in]
        n544 = call "LJM_eReadName.vi"("Handle In"=w1372, "Name"="DIO4_EF_READ_A_AND_RESET", "error in"=w1373) -> ("error out"=w1369:errorcluster)  [unwired: 10 in, 2 out]
        n545 = call <vilib>:"Add State(s) to Queue__JKI_lib_State_Machine.vi"("State(s) in (\"\")"=w1377) -> ("States Out"=w1376:string)  [unwired: 14 in]
      }
      frame "LJT4: Config" {
        w1382 = 1.0 ("element")
        w1383 = 10.0 ("element")
        w1384 = 0.0 ("element")
        w1386 = "DIO5_EF_ENABLE"
        w1387 = "DIO4_EF_ENABLE"
        # "Config T4 quadrature in\n(You can make a copy of, or modify, this frame)"
        n546 = Build Array(w1387, w1386, "DIO4_EF_INDEX", "DIO5_EF_INDEX", w1387, w1386) -> (w1385:string[])
        n547 = call "LabJack_FGV_T4.vi"("Operation(Read)"=enum16{"Write", "Read"}."Read" ("Operation"), "error in (no error)"=w1379) -> ("error out"=w1391:errorcluster, "Read data"=w1390:i32)  [unwired: 8 in]
        n548 = Build Array(w1384, w1384, w1383, w1383, w1382, w1382) -> (w1381:dbl[])
        n549 = call "LJM_eWriteNames.vi"("Handle In"=w1390, "aNames"=w1385, "aValuesIn"=w1381, "error in"=w1391) -> ("error out"=w1380:errorcluster)  [unwired: 9 in, 2 out]
        n550 = call <vilib>:"Add State(s) to Queue__JKI_lib_State_Machine.vi"("State(s) in (\"\")"=w1395) -> ("States Out"=w1394:string)  [unwired: 14 in]
      }
      frame "LJT4: Close" {
        # "Close T4 conncetion\n(You can make a copy of, or modify, this frame)"
        n551 = Unbundle By Name(w1397) -> ("Sys Status.T4"=w1399:bool)
        n552 = case shown="True" w1399 {
          tunnel: [w1405 w1411] -> w1401
          tunnel: w1400 -> [w1405 w1410]
          tunnel: w1397 -> [w1404 w1408]
          tunnel: [w1404 w1407] -> w1398
          frame False {
          }
          frame True {
            n553 = call "LabJack_FGV_T4.vi"("Operation(Read)"=enum16{"Write", "Read"}."Read" ("Operation"), "error in (no error)"=w1410) -> ("error out"=w1412:errorcluster, "Read data"=w1409:i32)  [unwired: 8 in]
            n554 = call "LJM_Close.vi"("error in"=w1412, "Handle"=w1409) -> ("error out"=w1411:errorcluster)  [unwired: 9 in]
            n555 = Bundle By Name(cluster=w1408, "Sys Status.T4"=FALSE) -> (w1407:T15)
          }
        }
        n556 = call <vilib>:"Add State(s) to Queue__JKI_lib_State_Machine.vi"("State(s) in (\"\")"=w1403) -> ("States Out"=w1402:string)  [unwired: 14 in]
      }
      frame "---------- USBCam ----------" {
        # "Template Separator\n(You can make a copy of, or modify, this frame)"
        n557 = call <vilib>:"Add State(s) to Queue__JKI_lib_State_Machine.vi"("State(s) in (\"\")"=w1418) -> ("States Out"=w1417:string)  [unwired: 14 in]
      }
      frame "USBCam: Initialize" {
        # "Template Separator\n(You can make a copy of, or modify, this frame)"
        n558 = call <vilib>:"IMAQdx Open Camera.vi"("error in"=w1430, "Session In"="CamSession In") -> ("error out"=w1423:errorcluster, "Session Out"=w1425:T4)  [unwired: 1 in, 7 out]
        n559 = call "IMAQ Create"("Image Name"="USB Image", "error in (no error)"=w1430) -> ("New Image"=w1421:T5, "error out"=w1431:errorcluster)  [unwired: 2 in, 1 out]
        "New Image" <- w1421
        n560 = call <vilib>:"IMAQdx Configure Grab.vi"("error in"=w1423, "Number of Buffers"=u32 5, "Session In"=w1425) -> ("error out"=w1422:errorcluster, "Session Out"=w1420:T4)  [unwired: 7 in]
        n561 = Bundle By Name(cluster=w1429, "IMAQ"=w1421, "USBCam"=w1420) -> (w1427:T15)
        n562 = Merge Errors(w1431, w1422) -> (w1428:errorcluster)
        n563 = case shown="No Error" w1428 {
          tunnel: w1427 -> [w1439 w1440]
          tunnel: [w1437 w1440] -> w1426
          frame No Error {
            n564 = Bundle By Name(cluster=w1439, "Sys Status.USB Cam"=TRUE) -> (w1437:T15)
            n565 = property on="Preview" class="Bool (strict)"("DisabledEnum"=T6."Enabled" ("Disabled")) -> ()  [unwired: 2 in, 2 out]
          }
          frame Error {
          }
        }
        n566 = call <vilib>:"Add State(s) to Queue__JKI_lib_State_Machine.vi"("State(s) in (\"\")"=w1435) -> ("States Out"=w1434:string)  [unwired: 14 in]
      }
      frame "USBCam: Grab" {
        # "Template Separator\n(You can make a copy of, or modify, this frame)"
        n567 = Unbundle By Name(w1443) -> ("IMAQ"=w1447:T5, "USBCam"=w1448:T4)
        n568 = call <vilib>:"IMAQdx Get Image2.vi"("Buffer Number Mode (Next)"=IMAQdx_Buffer_Number_Mode."Last New", "error in"=w1445, "Image In"=w1447, "Session In"=w1448) -> ("error out"=w1446:errorcluster, "Image Out"=w1442:T5)  [unwired: 4 in, 2 out]
        n569 = local write "Image"(w1442) -> ()
        n570 = call <vilib>:"Add State(s) to Queue__JKI_lib_State_Machine.vi"("State(s) in (\"\")"=w1450) -> ("States Out"=w1449:string)  [unwired: 14 in]
      }
      frame "USBCam: Close" {
        # "Close USB camra\n(You can make a copy of, or modify, this frame)"
        n571 = Unbundle By Name(w1453) -> ("IMAQ"=w1455:T5, "USBCam"=w1458:T4, "Sys Status.USB Cam"=w1451:bool)
        n572 = case shown="True" w1451 {
          tunnel: w1458 -> [_ w1470]
          tunnel: [w1462 w1468] -> w1457
          tunnel: w1456 -> [w1462 w1467]
          tunnel: w1455 -> [_ w1466]
          tunnel: w1453 -> [w1461 w1465]
          tunnel: [w1461 w1464] -> w1454
          frame False {
          }
          frame True {
            n573 = call <vilib>:"IMAQdx Close Camera.vi"("error in"=w1467, "Session In"=w1470) -> ("error out"=w1469:errorcluster)  [unwired: 9 out]
            n574 = call "Imaq Dispose"("Image"=w1466, "error in (no error)"=w1469) -> ("error out"=w1468:errorcluster)  [unwired: 4 in]
            n575 = Bundle By Name(cluster=w1465, "Sys Status.USB Cam"=FALSE) -> (w1464:T15)
          }
        }
        n576 = call <vilib>:"Add State(s) to Queue__JKI_lib_State_Machine.vi"("State(s) in (\"\")"=w1460) -> ("States Out"=w1459:string)  [unwired: 14 in]
      }
      frame "---------- Dialog ----------" {
        # "Template Separator\n(You can make a copy of, or modify, this frame)"
        n577 = call <vilib>:"Add State(s) to Queue__JKI_lib_State_Machine.vi"("State(s) in (\"\")"=w1475) -> ("States Out"=w1474:string)  [unwired: 14 in]
      }
      frame "Dialog: DataSaved" {
        # "Show data saved dialog\n(You can make a copy of, or modify, this frame)"
        n578 = Unbundle By Name(w1480) -> ("SaveFilePath"=w1479:path)
        n579 = Path To String(path=w1479) -> (string=w1477:string)
        n580 = Concatenate Strings("Data successfully save at " ("message"), w1477) -> (w1476:string)
        n581 = One Button Dialog(message=w1476) -> ()  [unwired: 1 in, 1 out]
        n582 = call <vilib>:"Add State(s) to Queue__JKI_lib_State_Machine.vi"("State(s) in (\"\")"=w1484) -> ("States Out"=w1483:string)  [unwired: 14 in]
      }
      frame "---------- New Category ----------" {
        # "Template Separator\n(You can make a copy of, or modify, this frame)"
        n583 = call <vilib>:"Add State(s) to Queue__JKI_lib_State_Machine.vi"("State(s) in (\"\")"=w1489) -> ("States Out"=w1488:string)  [unwired: 14 in]
      }
      frame "New Category: 1" {
        # "Your code here.\n(You can make a copy of, or modify, this frame)"
        n584 = call <vilib>:"Add State(s) to Queue__JKI_lib_State_Machine.vi"("State(s) in (\"\")"=w1494) -> ("States Out"=w1493:string)  [unwired: 14 in]
      }
      frame "New Category: 2" {
        # "Your code here.\n(You can make a copy of, or modify, this frame)"
        n585 = call <vilib>:"Add State(s) to Queue__JKI_lib_State_Machine.vi"("State(s) in (\"\")"=w1499) -> ("States Out"=w1498:string)  [unwired: 14 in]
      }
    }
  }
  n586 = while {
    tunnel: w26 -> [w1504]
    tunnel: [w1501] -> w25
    tunnel: w8 -> [w1500]
    stop <- w1502 stop-if-true
    # "Scan loop (both pre and follow)"
    n587 = event shown="[1] <3D profile scan pts>: User Event" {
      selector: w1504 -> [_ _ _]
      dyn-events: [_ _ _] -> w1501
      timeout: 10 -> [_ _ _]
      tunnel: [_ _ TRUE] -> w1502
      tunnel: w1500 -> [_ w1506 _]
      event Timeout {
        n588 = event-data() -> ()  [unwired: 1 in, 3 out]
      }
      event User Event {
        w1516 = "\r"
        n589 = event-data() -> ("3D profile scan pts"=w1509:cluster{"x(mm)":dbl, "y(mm)":dbl, "z(mm)":dbl}[])  [unwired: 1 in, 4 out]
        n590 = flat-sequence {
          tunnel: w1509 -> [w1522]
          tunnel: [w1522] -> w1508
          frame #0 {
            n591 = local write "Poll grbl position?"(FALSE ("Poll position")) -> ()
            n592 = Wait (ms)(milliseconds to wait=u32 100) -> ()  [unwired: 1 out]
          }
        }
        n593 = for {
          shift-right: [w1528] -> w1511
          shift-left: errorcluster {"status"=FALSE, "code"=0, "source"=""} ("error out") -> [w1530]
          tunnel: w1508 -> [w1527] mode=indexing
          stop <- w1528 stop-if-true
          n594 = Unbundle By Name(w1527) -> ("x(mm)"=w1526:dbl, "y(mm)"=w1525:dbl, "z(mm)"=w1524:dbl)
          n595 = Not A Number/Path/Refnum?(number/path/refnum=w1524) -> (NaN/Path/Refnum?=w1529:bool)
          n596 = case shown="False" w1529 {
            tunnel: w1530 -> [w1535 w1537]
            tunnel: [w1534 w1537] -> w1528
            tunnel: w1526 -> [w1533 _]
            tunnel: w1525 -> [w1532 _]
            tunnel: w1524 -> [w1531 _]
            frame False {
              # "if z not NaN, send"
              n597 = call "Go to Position.vi"("X (mm)"=w1533, "Y (mm)"=w1532, "Z (mm)"=w1531, "Wait for finish? (T)"=FALSE, "error in (no error)"=w1535) -> ("error out"=w1534:errorcluster)  [unwired: 10 in]
            }
            frame True {
              # "if z is NaN, do nothing"
            }
          }
        }
        n598 = while {
          shift-right: [w1546] -> w1507
          shift-left: w1511 -> [w1547]
          i -> [w1541]
          stop <- w1538 stop-if-true
          n599 = Greater?(x=w1541, y=500) -> (0:w1539:bool)
          n600 = call "Get Status.vi"("error in (no error)"=w1547) -> ("Status"=w1545:T9, "error out"=w1546:errorcluster)  [unwired: 10 in, 3 out]
          n601 = Wait (ms)(milliseconds to wait=u32 100) -> ()  [unwired: 1 out]
          n602 = Equal?(x=Status."Idle" ("Status"), y=w1545) -> (x = y?=w1542:bool)
          n603 = Or(x=w1542, y=w1539) -> (x .or. y?=w1538:bool)
        }
        n604 = Generate User Event(user event=w1506, event data cluster=TRUE ("event data"), error in=w1507) -> ()  [unwired: 1 in, 2 out]
        n605 = Concatenate Strings("$120=500" ("string"), w1516) -> (w1515:string)
        n606 = Concatenate Strings("$121=200" ("string"), w1516) -> (w1514:string)
        n607 = Concatenate Strings("$122=500" ("string"), w1516) -> (w1513:string)
        n608 = flat-sequence {
          tunnel: w1507 -> [_]
          frame #0 {
            n609 = local write "Poll grbl position?"(TRUE ("Poll position")) -> ()
          }
        }
        n610 = Build Array(w1515, w1514, w1513) -> (w1512:string[])
        n611 = for {
          tunnel: w1507 -> [w1549]
          tunnel: w1512 -> [w1548] mode=indexing
          n612 = call "Send-Receive Serial Port.vi"("Data to write"=w1548, "error in (no error)"=w1549) -> ()  [unwired: 12 in, 2 out]
        }
      }
      event User Event {
        n613 = event-data() -> ()  [unwired: 1 in, 5 out]
      }
    }
  }
  n614 = while {
    tunnel: w46 -> [w1554]
    tunnel: [w1553] -> w44
    tunnel: w38 -> [w1552]
    stop <- w1551 stop-if-true
    # "3D profile data aquisition loop"
    n615 = event shown="[1] <Start Range Finder>: User Event" {
      selector: w1554 -> [_ _]
      dyn-events: [_ _] -> w1553
      timeout: 5 -> [_ _]
      tunnel: w1552 -> [w1557 w1563]
      tunnel: [w1556 w1559] -> w1551
      event Timeout {
        n616 = event-data() -> ()  [unwired: 1 in, 3 out]
        n617 = Get Queue Status(queue=w1557) -> (error out=w1556:errorcluster)  [unwired: 2 in, 7 out]
      }
      event User Event {
        n618 = event-data() -> ()  [unwired: 1 in, 1 out]
        n619 = local read "Range Finder COM"() -> (w1565:refnum<visa-resource-name>)
        n620 = call "LabJack_FGV_T4.vi"("Operation(Read)"=enum16{"Write", "Read"}."Read" ("Operation")) -> ("error out"=w1561:errorcluster, "Read data"=w1560:i32)  [unwired: 9 in]
        n621 = while {
          tunnel: w1565 -> [w1591]
          shift-right: [w1585] -> w1559
          shift-left: errorcluster {"status"=FALSE, "code"=0, "source"=""} ("error in (no error)") -> [w1573]
          tunnel: w1563 -> [w1582]
          tunnel: w1561 -> [w1575]
          tunnel: w1560 -> [w1576]
          shift-right: [w1571] -> _
          shift-left: 0.0 ("relative seconds") -> [w1570]
          i -> [w1569]
          stop <- w1588 stop-if-true
          # "3D profile aquisition loop"
          n622 = VISA Read(VISA resource name=w1591, byte count=4, error in (no error)=w1573) -> (read buffer=w1579:string, error out=w1572:errorcluster)  [unwired: 2 out]
          "read buffer" <- w1579
          n623 = Quotient & Remainder(x=w1569, y=10) -> (x-y*floor(x/y)=w1567:i32)  [unwired: 1 out]
          n624 = String Length(string=w1579) -> (length=w1589:i32)
          n625 = call "LJM_eReadName.vi"("Handle In"=w1576, "Name"="DIO4_EF_READ_A_F", "error in"=w1575) -> ("Value"=w1584:dbl, "error out"=w1574:errorcluster)  [unwired: 10 in, 1 out]
          "X encoder count" <- w1584
          n626 = Equal To 0?(x=w1567) -> (x = 0?=w1566:bool)
          n627 = Equal?(x=w1589, y=3) -> (x = y?=w1577:bool)
          n628 = call <vilib>:"High Resolution Relative Seconds.vi"() -> ("relative seconds"=w1571:dbl)
          n629 = Multiply(x=w1584, y=0.0025) -> (x*y=w1581:dbl)
          "X (mm)" <- w1581
          n630 = case shown="True" w1566 {
            tunnel: w1571 -> [_ w1596]
            tunnel: w1570 -> [_ w1595]
            frame False {
            }
            frame True {
              n631 = Subtract(x=w1596, y=w1595) -> (x-y=w1594:dbl)
              n632 = Multiply(x=w1594, y=1000.0) -> (x*y=→"dt polling (ms)":dbl)
            }
          }
          n633 = case shown="False" w1577 {
            tunnel: w1579 -> [_ w1604]
            tunnel: [0.0 ("Distance(mm)") w1603] -> w1578
            frame False {
            }
            frame True {
              n634 = call "BinaryToMilimeter.vi"("Hex string"=w1604) -> ("Distance(mm)"=w1603:dbl)  [unwired: 10 in]
            }
          }
          "Z Distance(mm)" <- w1578
          n635 = Merge Errors(w1572, w1574) -> (w1585:errorcluster)
          n636 = case shown="True" w1577 {
            tunnel: w1582 -> [_ w1601]
            tunnel: w1581 -> [_ w1599]
            tunnel: w1578 -> [_ w1598]
            frame False {
            }
            frame True {
              n637 = Bundle(w1599, 0.0, "Distance(mm)"=w1598) -> (w1600:cluster{dbl, dbl, "Distance(mm)":dbl})  [unwired: 1 in]
              n638 = Enqueue Element(queue=w1601, element=w1600) -> ()  [unwired: 2 in, 3 out]
            }
          }
          n639 = Or(x=w1585, y="AccuRangeLoopStopFlag") -> (x .or. y?=w1588:bool)
        }
        "3D scan" <- w1559
      }
    }
  }
  n640 = while {
    tunnel: w13 -> [w1608]
    stop <- w1606 stop-if-true
    # "Waveform display loop"
    n641 = Wait (ms)(milliseconds to wait=u32 20) -> ()  [unwired: 1 out]
    n642 = Wait on Notification(notifier=w1608) -> (notification=→"PPIX intensity trace":dbl, error out=w1606:errorcluster)  [unwired: 3 in, 2 out]
  }
  n643 = while {
    tunnel: w22 -> [w1613]
    tunnel: w13 -> [w1611]
    tunnel: [w1610] -> w17
    tunnel: w4 -> [w1609]
    stop <- w1612 stop-if-true
    # "FLIm DAQ"
    n644 = event shown="[0] <Start FLIm>: User Event" {
      selector: w1613 -> [_ _ _]
      dyn-events: [_ _ _] -> w1610
      timeout: 5 -> [_ _ _]
      tunnel: [FALSE FALSE TRUE] -> w1612
      tunnel: w1611 -> [w1624 _ _]
      tunnel: w1609 -> [w1622 _ _]
      event User Event {
        n645 = event-data() -> ("Time"=→"LocationPollingStart":u32)  [unwired: 1 in, 4 out]
        n646 = Flush Queue(queue=w1622) -> (queue out=w1617:refnum<queue>)  [unwired: 1 in, 2 out]
        n647 = call "LabJack_FGV_T4.vi"("Operation(Read)"=enum16{"Write", "Read"}."Read" ("Operation")) -> ("error out"=w1620:errorcluster, "Read data"=w1619:i32)  [unwired: 9 in]
        n648 = Tick Count (ms)() -> (millisecond timer value=w1616:u32)
        n649 = while {
          tunnel: w1624 -> [w1649]
          shift-right: [w1635] -> _
          shift-left: 0.0 ("relative seconds") -> [w1648]
          tunnel: w1617 -> [w1644]
          tunnel: w1620 -> [w1629]
          tunnel: w1619 -> [w1642]
          tunnel: w1616 -> [w1626]
          stop <- w1636 stop-if-true
          n650 = call <vilib>:"High Resolution Relative Seconds.vi"() -> ("relative seconds"=w1635:dbl)
          n651 = Subtract(x=w1635, y=w1648) -> (x-y=w1634:dbl)
          n652 = call <userlib>:"Tick Count (ms)__ogtk.vi"("error in (no error)"=w1629) -> ("error out"=w1628:errorcluster, "millisecond timer value"=w1627:u32)  [unwired: 9 in]
          n653 = Multiply(x=w1634, y=1000.0) -> (x*y=w1632:dbl)
          n654 = local write "dt polling (ms)"(w1632) -> ()
          n655 = Subtract(x=w1627, y=w1626) -> (x-y=w1625:u32)
          n656 = call "LJM_eReadName.vi"("Handle In"=w1642, "Name"="DIO4_EF_READ_A_F", "error in"=w1628) -> ("Value"=w1630:dbl, "error out"=w1646:errorcluster)  [unwired: 10 in, 1 out]
          n657 = local write "X encoder count"(w1630) -> ()
          n658 = Multiply(x=w1630, y=0.0025) -> (x*y=w1631:dbl)
          n659 = local write "X (mm)"(w1631) -> ()
          n660 = Send Notification(notification=w1625, notifier=w1649) -> (error out=w1647:errorcluster)  [unwired: 1 in, 1 out]
          n661 = Bundle(w1625, w1631) -> (w1641:cluster{u32, dbl})  [unwired: 1 in]
          n662 = Enqueue Element(queue=w1644, element=w1641) -> (error out=w1643:errorcluster)  [unwired: 2 in, 2 out]
          n663 = Merge Errors(w1647, w1646, w1643) -> (w1637:errorcluster)
          n664 = Not(x="FollowScan") -> (.not. x?=w1638:bool)
          n665 = Or(x=w1638, y=w1637) -> (x .or. y?=w1636:bool)
        }
      }
      event Timeout {
        n666 = event-data() -> ()  [unwired: 1 in, 3 out]
      }
      event User Event {
        n667 = event-data() -> ()  [unwired: 1 in, 5 out]
      }
    }
  }
  n668 = local write "Poll grbl position?"(TRUE) -> ()
  n669 = local write "Preview"(FALSE ("Preview")) -> ()
  n670 = property on="Preview" class="Bool (strict)"("DisabledEnum"=T6."Disabled and Grayed Out" ("Disabled")) -> ()  [unwired: 2 in, 2 out]
  n671 = Unregister For Events(event registration refnum=w17, error in=w9) -> (error out=w16:errorcluster)
  n672 = Release Notifier(notifier=w13, error in (no error)=w9) -> (error out=w20:errorcluster)  [unwired: 1 in, 2 out]
  n673 = Unregister For Events(event registration refnum=w10, error in=w9) -> (error out=w7:errorcluster)
  n674 = Unregister For Events(event registration refnum=w44, error in=w43) -> (error out=w45:errorcluster)
  n675 = Unregister For Events(event registration refnum=w25, error in=w9) -> (error out=w24:errorcluster)
  n676 = Destroy User Event(user event=w8, error in=w7) -> (error out=w2:errorcluster)
  n677 = Release Queue(queue=w38, error in (no error)=w9) -> (error out=w40:errorcluster)  [unwired: 1 in, 2 out]
  n678 = Destroy User Event(user event=w29, error in=w45) -> (error out=w33:errorcluster)
  n679 = Destroy User Event(user event=w19, error in=w24) -> (error out=w23:errorcluster)
  n680 = Destroy User Event(user event=w1, error in=w9) -> (error out=w14:errorcluster)
  n681 = Merge Errors(w2, w40, w33, w9, w23, w20, w18, w16, w14) -> (w39:errorcluster)
  n682 = call <vilib>:"Simple Error Handler.vi"("error in (no error)"=w39) -> ()  [unwired: 4 in, 5 out]
